vi "LR5_code.vi"(7 "data in":string, 8 "error in (no error)":errorcluster, 9 "Image Dst":T1) -> (0 "error out":errorcluster, 2 "data out":string)   [LabVIEW 2019]
uses:
  <vilib>/vision/Image Controls.llb/IMAQ Image.ctl
  Stage_var.vi
  Init_var.vi
  Color_num_var.vi
  Timer.vi
  Global_count_var.vi
  Camera_angle.vi
  Arm_stage_var.vi
  Mashina_podyehala.vi
  Ball_num_var.vi
  Completed_var.vi
  Sequence_var.vi
  Scanned.vi
  <vilib>/vision/NI_Vision_Development_Module.lvlib
  Simulated Robot/Simulation SubVIs/Simulation SubVIs.lvlib
panel:
  out "Left":dbl(slide)
  out "Right":dbl(slide) scale=0.0..1.0
  out "ForwR":dbl(slide) scale=0.0..1.0
  out "ForwL":dbl(slide) scale=0.0..1.0
  out "ForwardRight Distance (m)":dbl
  out "ForwardLeft Distance (m)":dbl
  out "Right Distance (m)":dbl
  out "Left Distance (m)":dbl
  in  "Start":bool
  out "Stage":u32
  out "Ball num":dbl
  out "Color now":dbl
  out "Arm stage":dbl
  out "Image":T1(plugin-control)
  out "Sequence":dbl[](array[numeric])
  out "Scanned":bool
  out "Completed":bool
  out "Performing...":u8(slide) scale=4.0..107.0
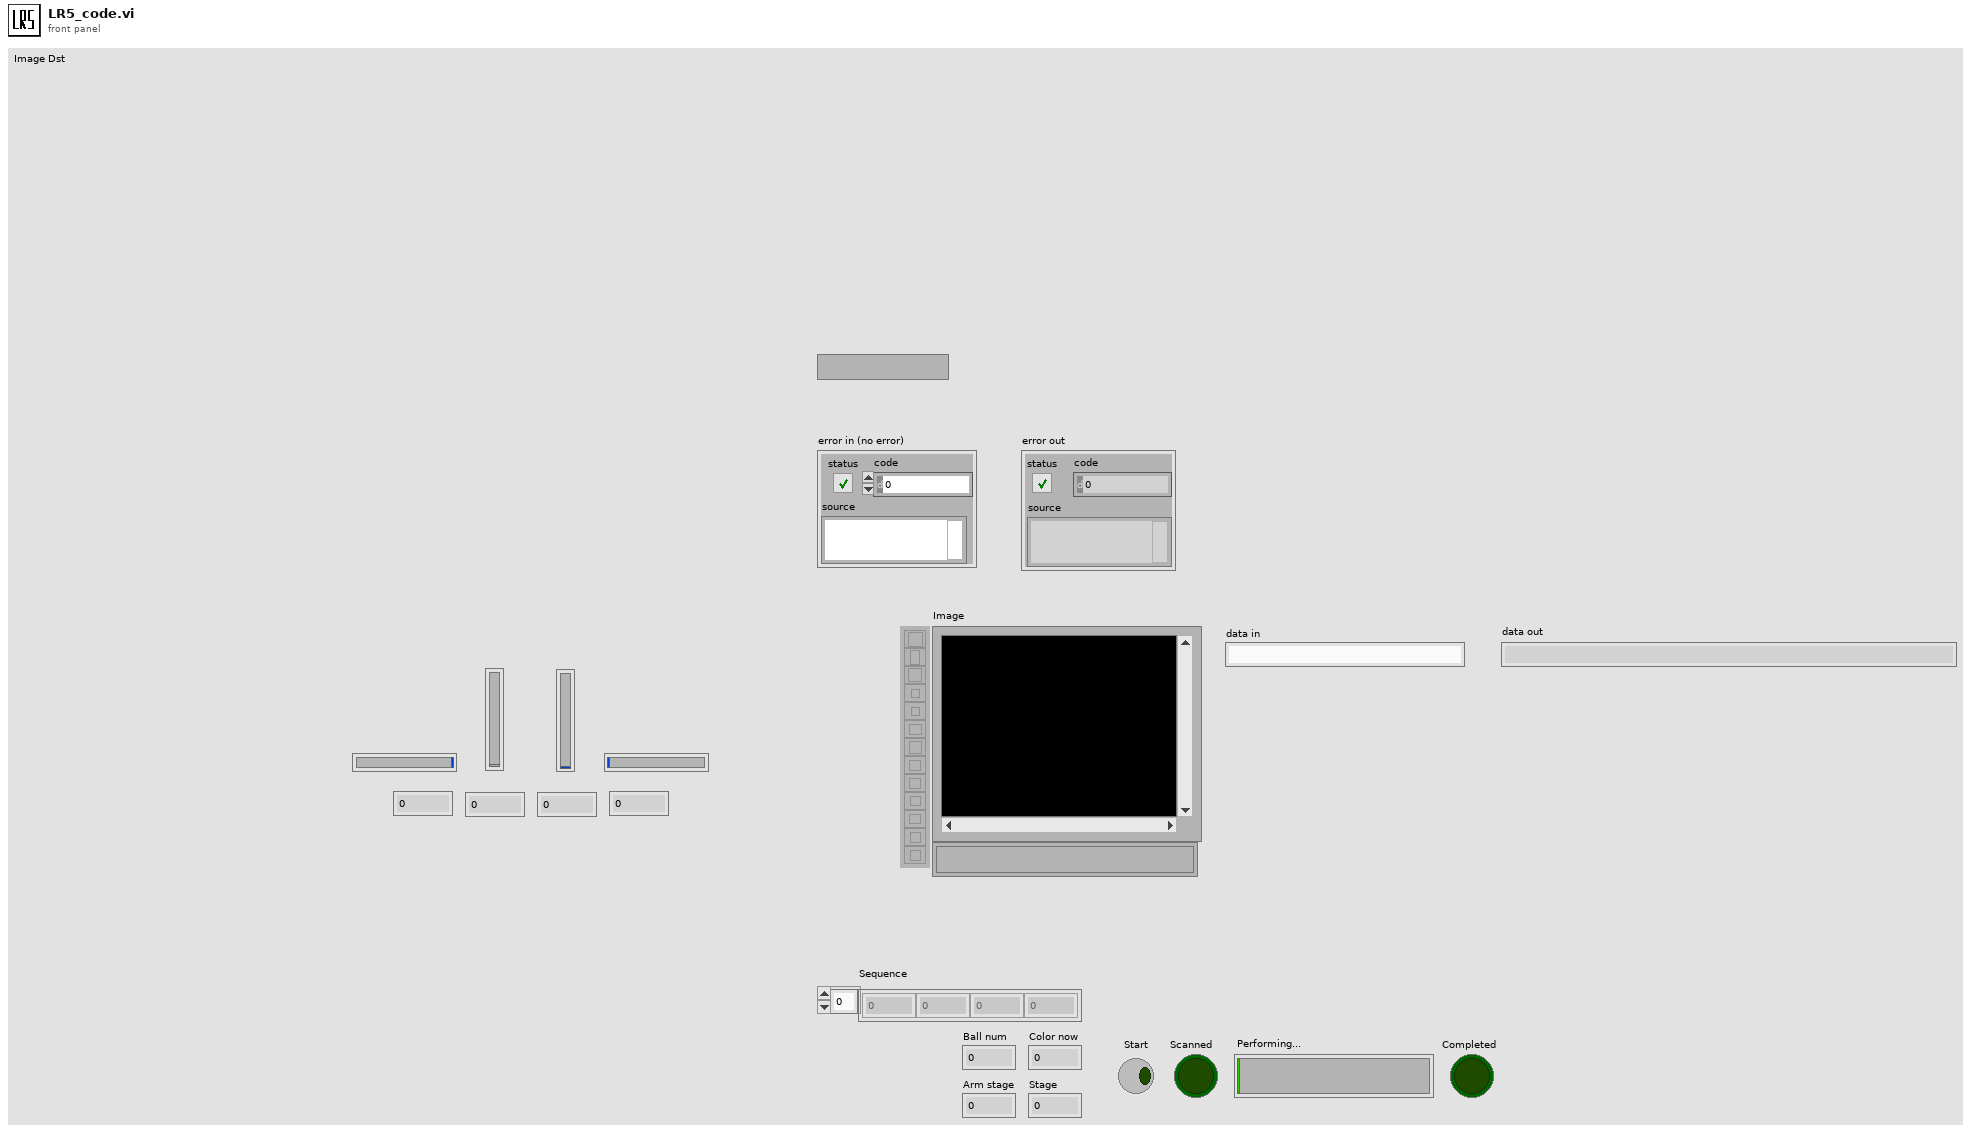
[diagram p1: front panel]
types:
  T1 = typedef "IMAQ Image.ctl" = refnum<image>
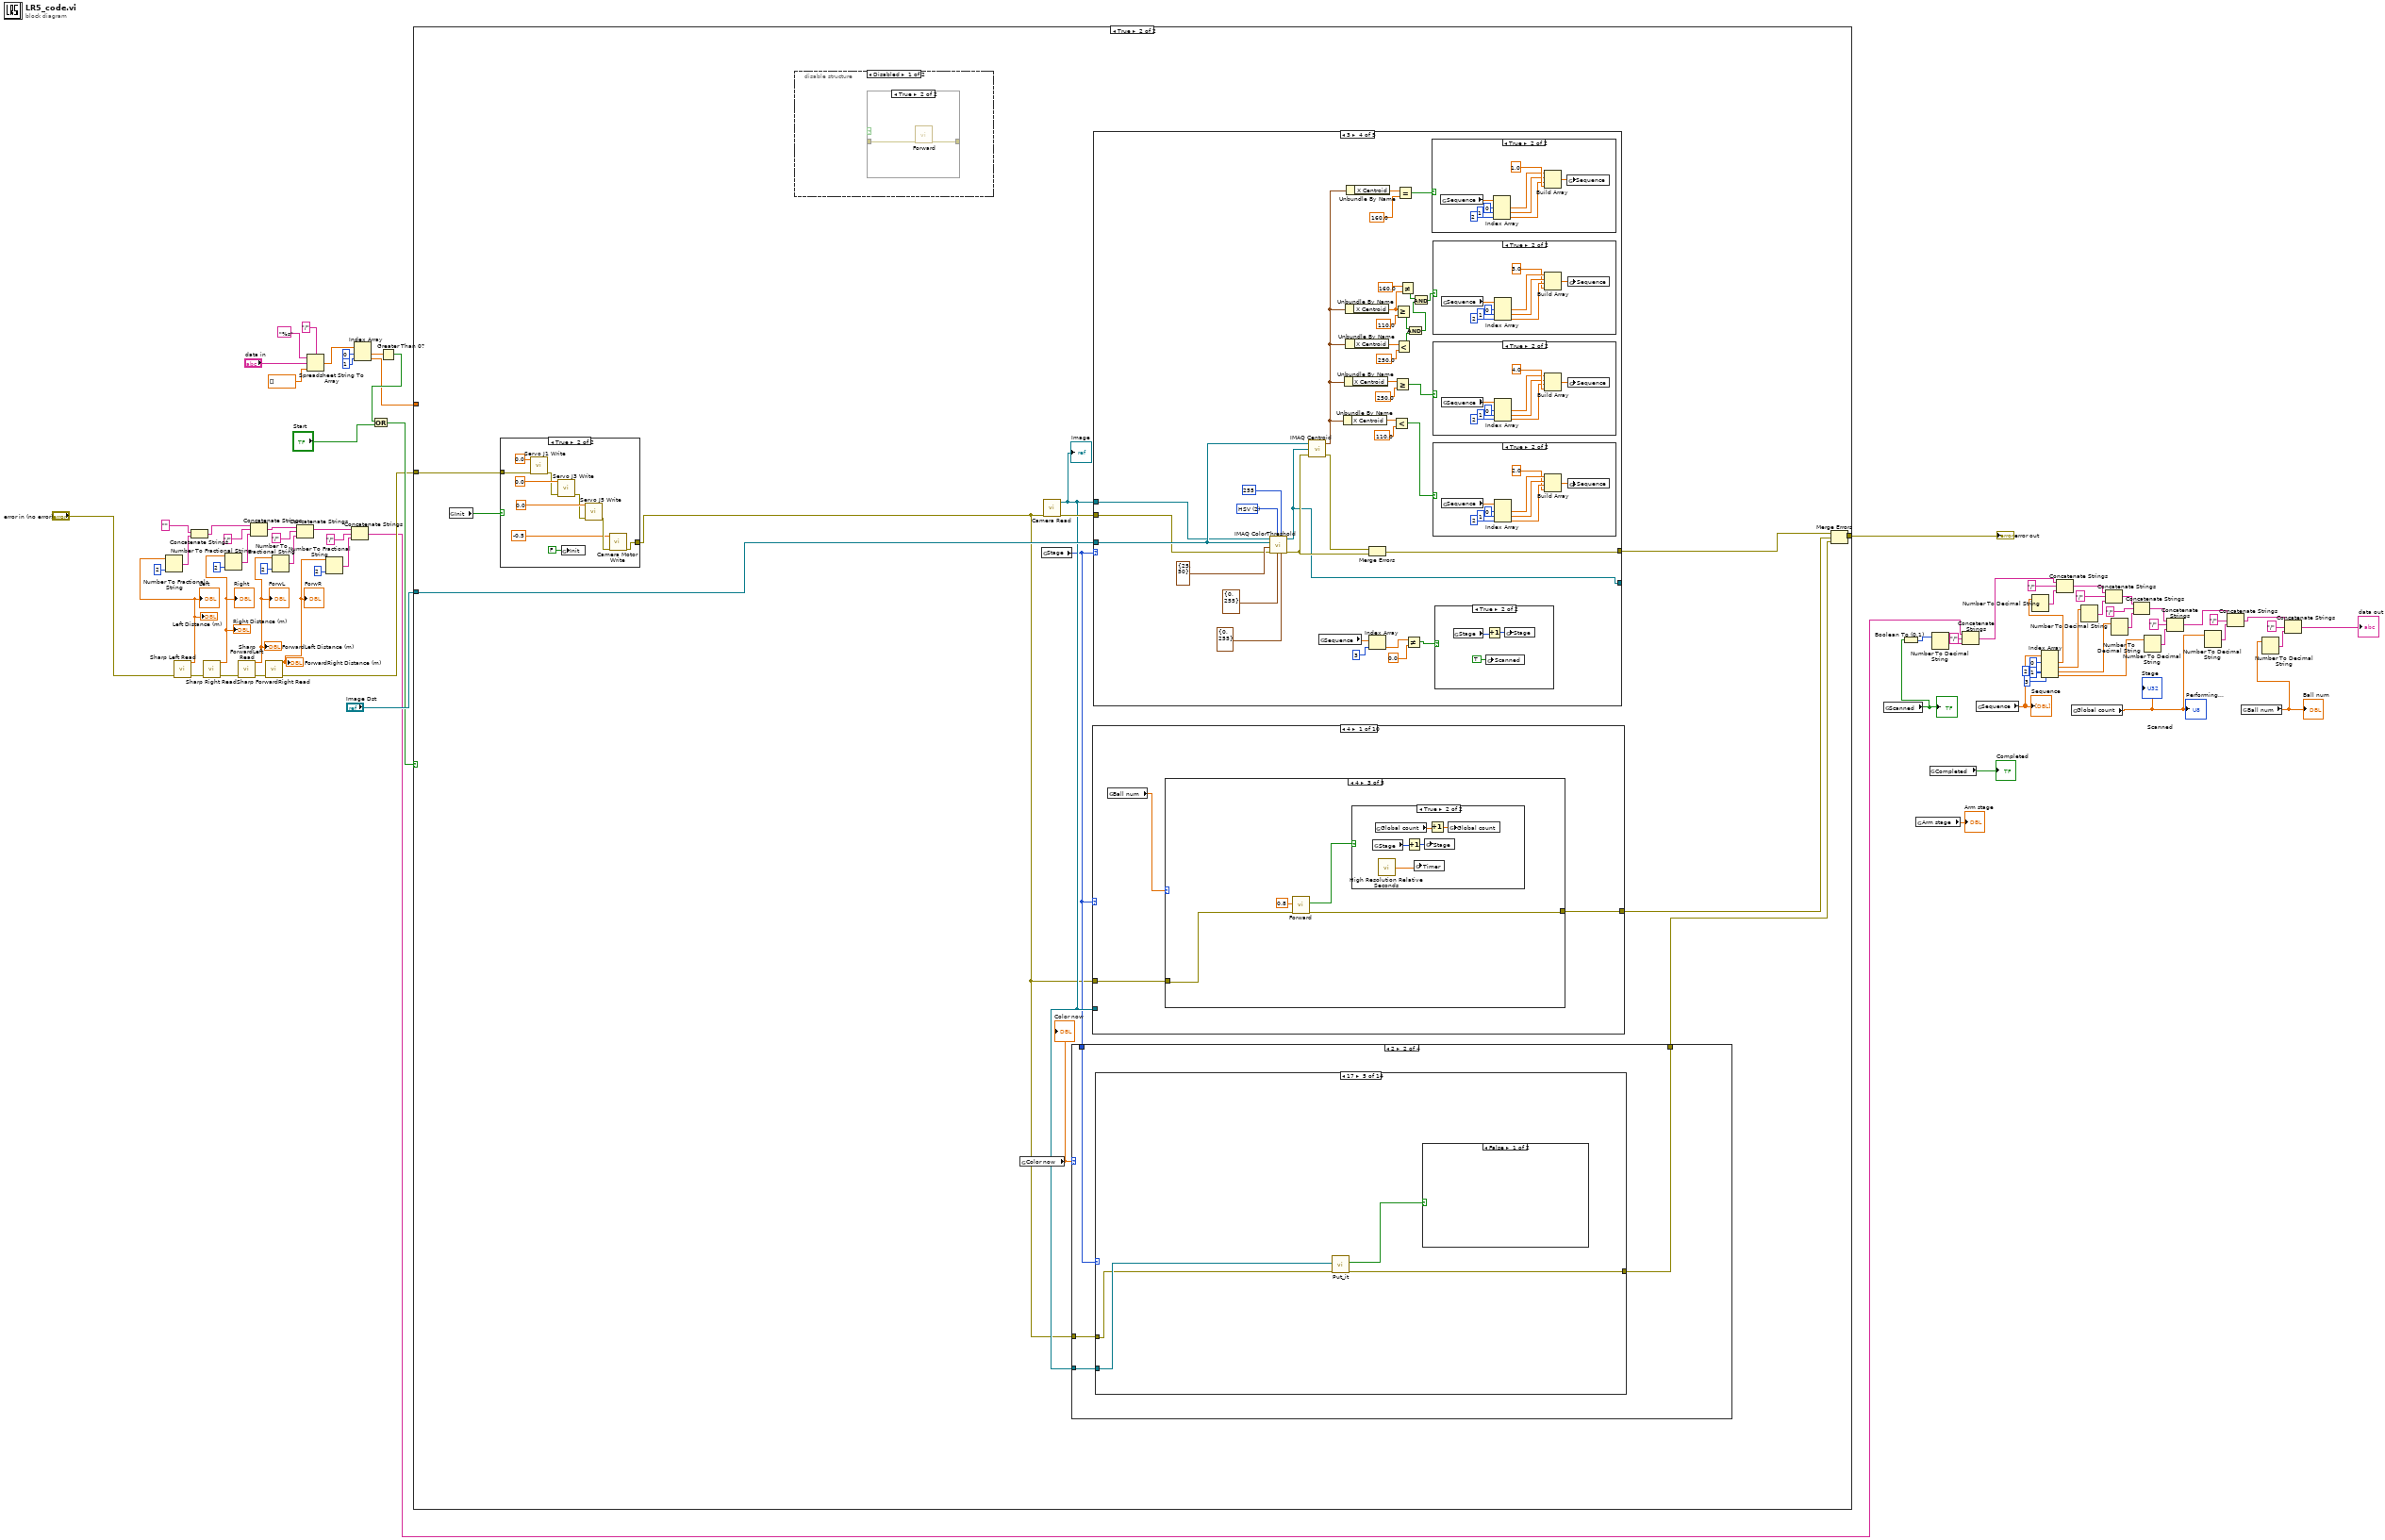
[diagram p0: block diagram]
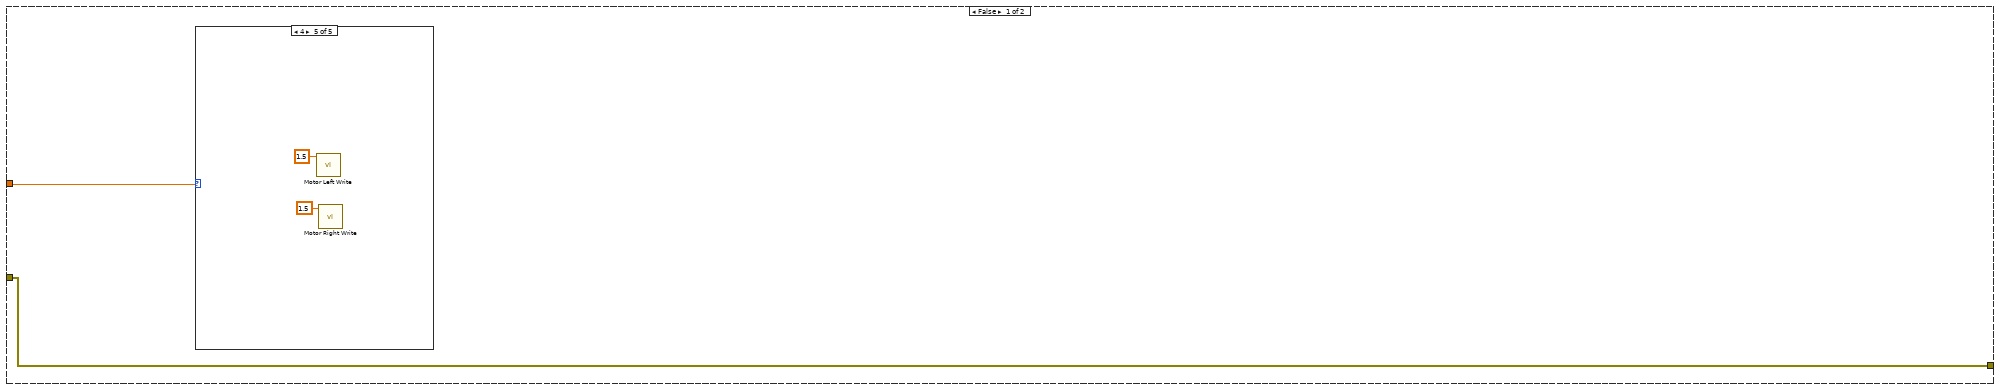
[diagram p2: hidden frame]
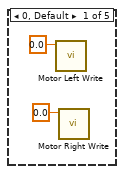
[diagram p3: hidden frame]
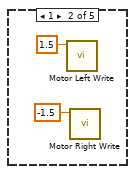
[diagram p4: hidden frame]
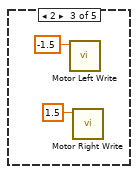
[diagram p5: hidden frame]
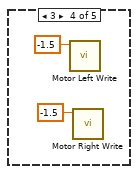
[diagram p6: hidden frame]
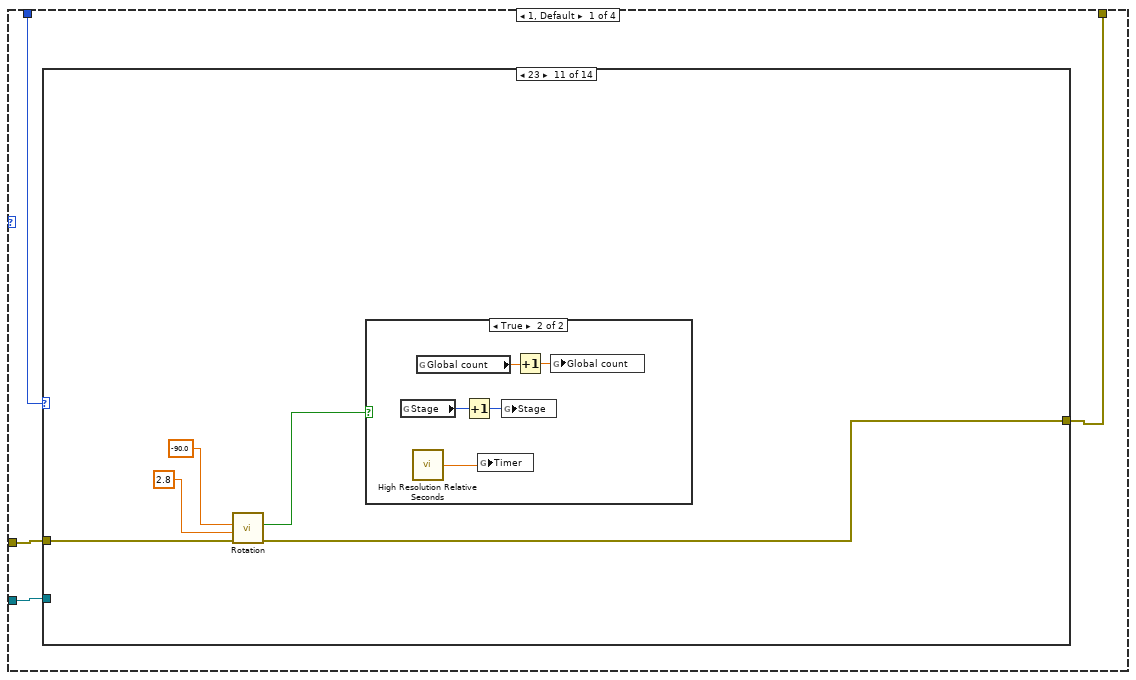
[diagram p7: hidden frame]
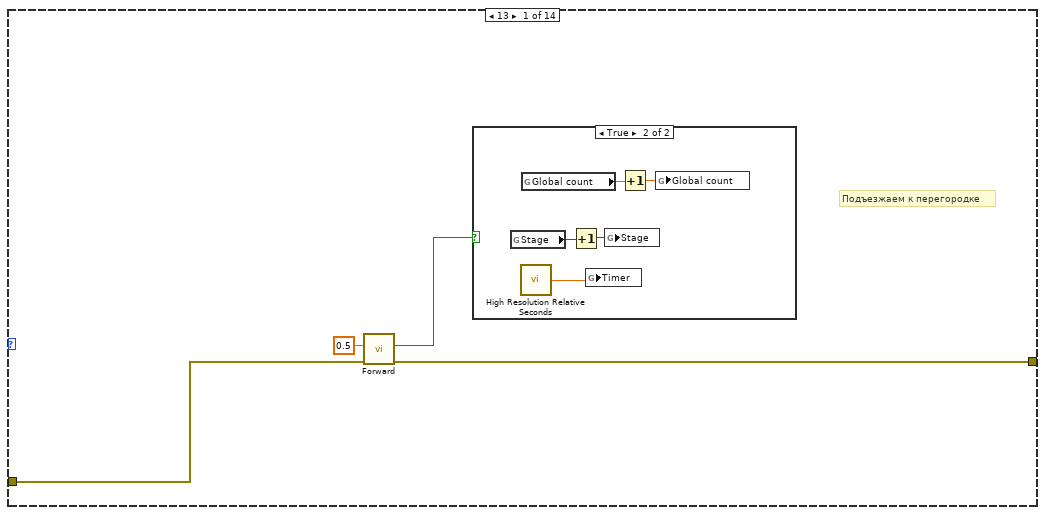
[diagram p8: hidden frame]
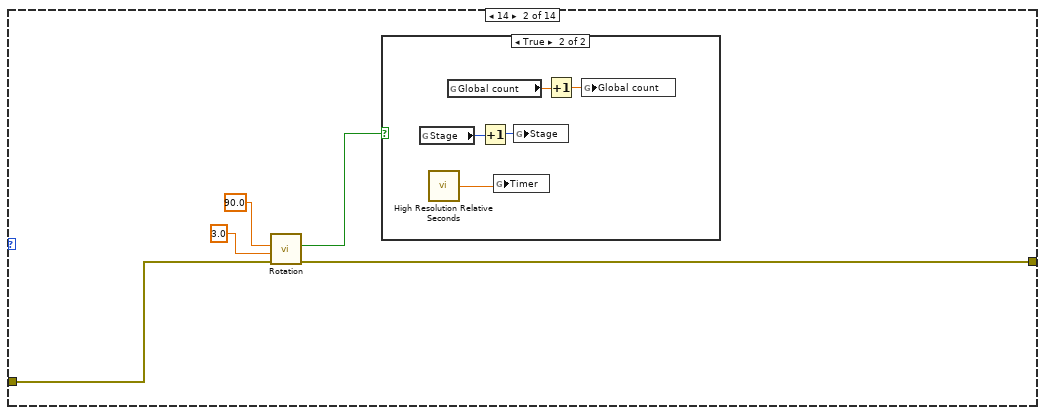
[diagram p10: hidden frame]
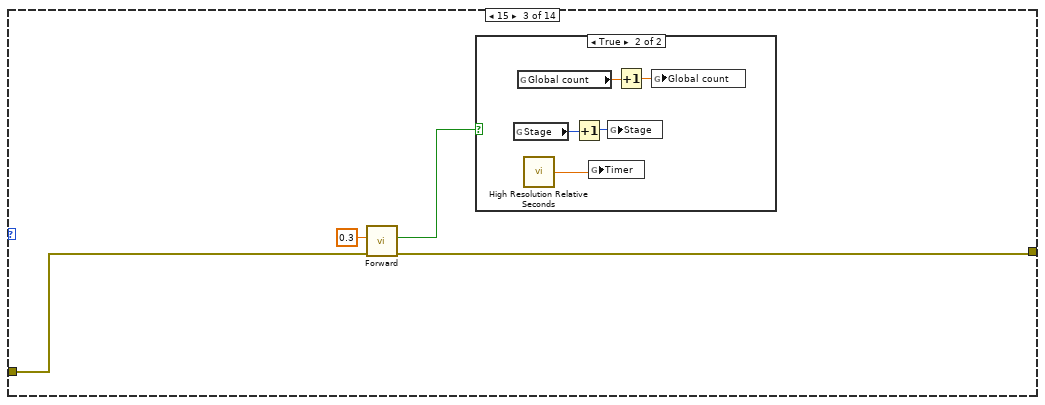
[diagram p12: hidden frame]
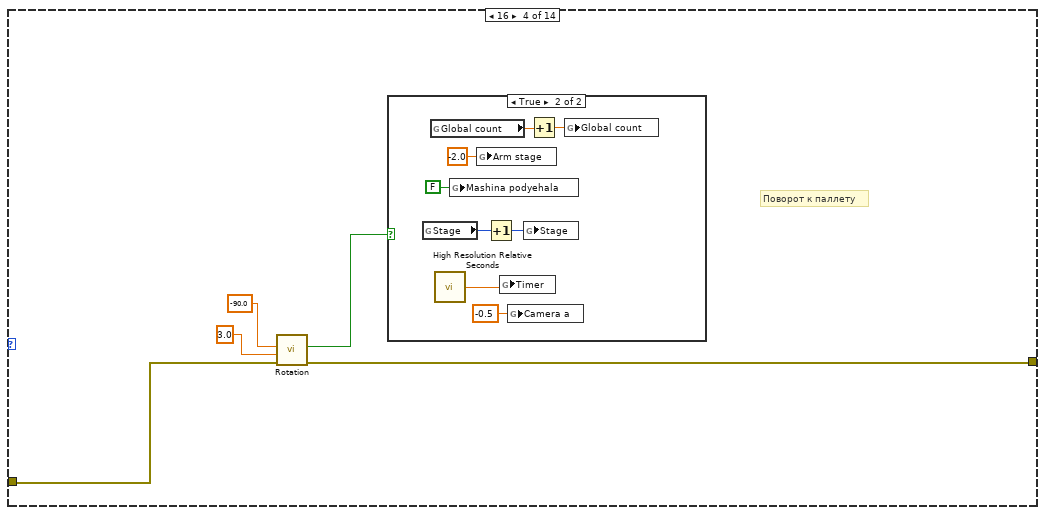
[diagram p14: hidden frame]
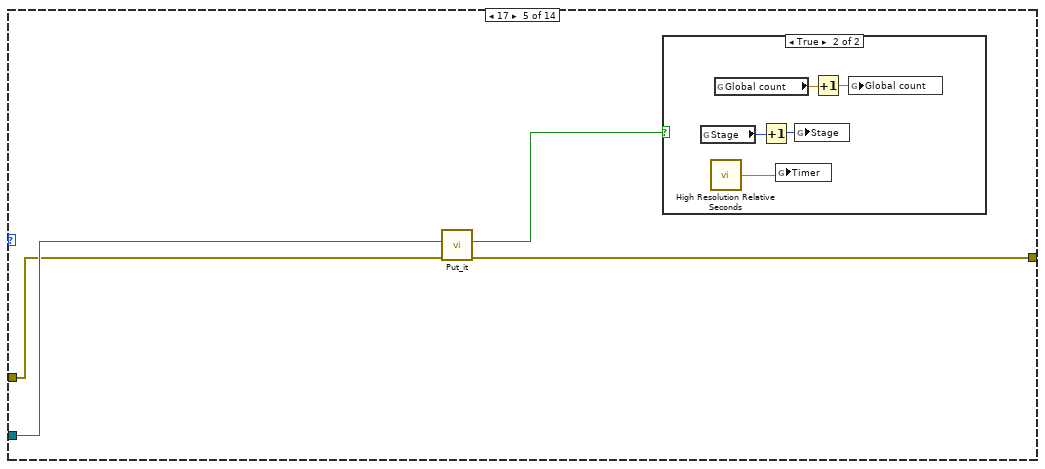
[diagram p16: hidden frame]
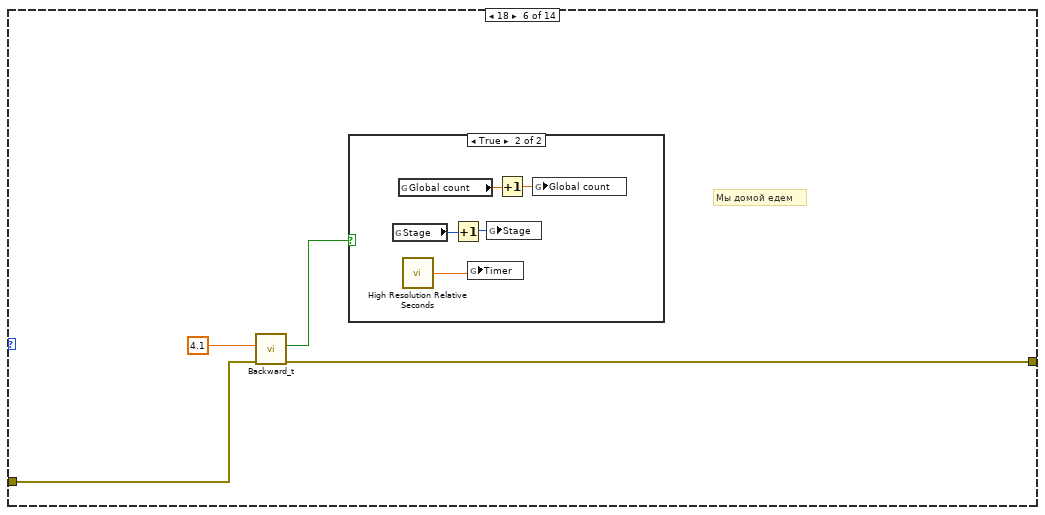
[diagram p18: hidden frame]
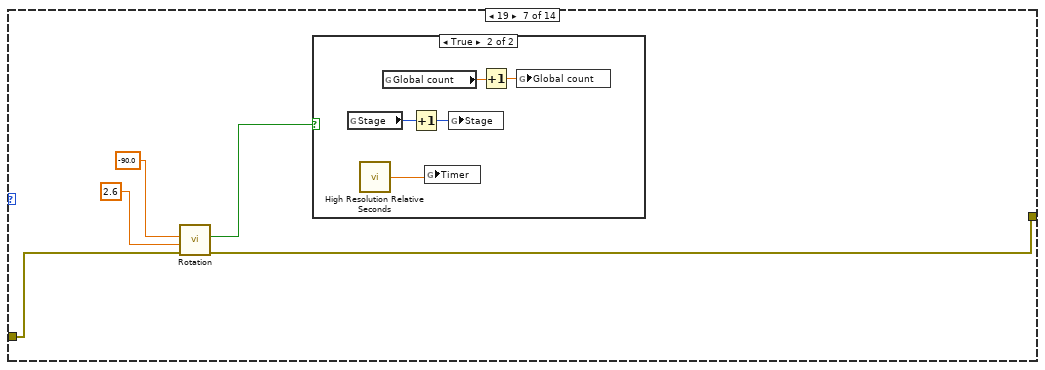
[diagram p20: hidden frame]
diagram:
  n1 = call "Sharp Left Read.vi"("error in (no error)"="error in (no error)") -> ("error out"=w59:errorcluster, "Left Distance (m)"=w52:dbl)  [unwired: 9 in]
  "Left Distance (m)" <- w52
  "Left" <- w52
  n2 = Number To Fractional String(number=w52, precision (6)=i16 2) -> (F-format string=w51:string)  [unwired: 2 in]
  n3 = Concatenate Strings("" ("string"), w51) -> (w41:string)
  n4 = call "Sharp Right Read.vi"("error in (no error)"=w59) -> ("error out"=w58:errorcluster, "Right Distance (m)"=w48:dbl)  [unwired: 9 in]
  "Right Distance (m)" <- w48
  "Right" <- w48
  n5 = Number To Fractional String(number=w48, precision (6)=i16 2) -> (F-format string=w50:string)  [unwired: 2 in]
  n6 = call "Sharp ForwardLeft Read.vi"("error in (no error)"=w58) -> ("error out"=w57:errorcluster, "ForwardLeft Distance (m)"=w45:dbl)  [unwired: 9 in]
  "ForwardLeft Distance (m)" <- w45
  "ForwL" <- w45
  n7 = Concatenate Strings(w41, "/" ("string"), w50) -> (w39:string)
  n8 = call "Sharp ForwardRight Read.vi"("error in (no error)"=w57) -> ("error out"=w55:errorcluster, "ForwardRight Distance (m)"=w42:dbl)  [unwired: 9 in]
  "ForwardRight Distance (m)" <- w42
  "ForwR" <- w42
  n9 = Number To Fractional String(number=w45, precision (6)=i16 2) -> (F-format string=w46:string)  [unwired: 2 in]
  n10 = Concatenate Strings(w39, "/" ("string"), w46) -> (w37:string)
  n11 = Spreadsheet String To Array(delimiter (Tab)="/", format string="%s", spreadsheet string="data in", array type (2D Dbl)=dbl[] []) -> (array=w71:dbl[])
  n12 = Number To Fractional String(number=w42, precision (6)=i16 2) -> (F-format string=w43:string)  [unwired: 2 in]
  n13 = Concatenate Strings(w37, "/" ("string"), w43) -> (w10:string)
  n14 = Index Array(array=w71, index #1=0 ("index"), index #2=1 ("index")) -> (element #1=w64:dbl, element #2=w62:dbl)
  n15 = Greater Than 0?(x=w64) -> (x > 0?=w63:bool)
  n16 = Or(x=w63, y="Start") -> (x .or. y?=w70:bool)
  n17 = case shown="True" w70 {
    tunnel: w55 -> [w77 w99]
    tunnel: [w77 w95] -> w75
    tunnel: "Image Dst" -> [_ w93]
    tunnel: w62 -> [w76 _]
    frame False {
      n18 = case shown="4" w76 {
        frame 0, Default {
          n19 = call "Motor Left Write.vi"("left motor ccw velocity (rad/s)"=0.0) -> ()  [unwired: 10 in, 1 out]
          n20 = call "Motor Right Write.vi"("right motor ccw velocity (rad/s)"=0.0) -> ()  [unwired: 10 in, 1 out]
        }
        frame 1 {
          n21 = call "Motor Left Write.vi"("left motor ccw velocity (rad/s)"=1.5) -> ()  [unwired: 10 in, 1 out]
          n22 = call "Motor Right Write.vi"("right motor ccw velocity (rad/s)"=-1.5) -> ()  [unwired: 10 in, 1 out]
        }
        frame 2 {
          n23 = call "Motor Left Write.vi"("left motor ccw velocity (rad/s)"=-1.5) -> ()  [unwired: 10 in, 1 out]
          n24 = call "Motor Right Write.vi"("right motor ccw velocity (rad/s)"=1.5) -> ()  [unwired: 10 in, 1 out]
        }
        frame 3 {
          n25 = call "Motor Left Write.vi"("left motor ccw velocity (rad/s)"=-1.5) -> ()  [unwired: 10 in, 1 out]
          n26 = call "Motor Right Write.vi"("right motor ccw velocity (rad/s)"=-1.5) -> ()  [unwired: 10 in, 1 out]
        }
        frame 4 {
          n27 = call "Motor Left Write.vi"("left motor ccw velocity (rad/s)"=1.5) -> ()  [unwired: 10 in, 1 out]
          n28 = call "Motor Right Write.vi"("right motor ccw velocity (rad/s)"=1.5) -> ()  [unwired: 10 in, 1 out]
        }
      }
    }
    frame True {
      n29 = global read "Init_var.vi" "Init"() -> (w98:bool)
      n30 = case shown="True" w98 {
        tunnel: w99 -> [w1006 w1009]
        tunnel: [w1006 w1007] -> w88
        frame False {
        }
        frame True {
          n31 = call "Servo J1 Write.vi"("error in (no error)"=w1009, "J1 Position (m)"=0.0) -> ("error out"=w1014:errorcluster)  [unwired: 9 in]
          n32 = call "Servo J3 Write.vi"("error in (no error)"=w1014, "J3 Position (m)"=0.0) -> ("error out"=w1013:errorcluster)  [unwired: 9 in]
          n33 = global write "Init_var.vi" "Init"(FALSE ("Init")) -> ()
          n34 = call "Servo J5 Write.vi"("error in (no error)"=w1013, "J5 Position (m)"=0.0) -> ("error out"=w1012:errorcluster)  [unwired: 9 in]
          n35 = call "Camera Motor Write.vi"("error in (no error)"=w1012, "Camera Position (rad)"=-0.5) -> ("error out"=w1007:errorcluster)  [unwired: 9 in]
        }
      }
      n36 = disable-structure shown="Disabled" {
        frame Disabled {
          n37 = case shown="True" w1321 {
            tunnel: [w1322 w1324] -> w1320
            tunnel: [w1322 w1323] -> _
            frame False {
            }
            frame True {
              n38 = call "Forward.vi"("error in (no error)"=w1324) -> ("error out"=w1323:errorcluster)  [unwired: 9 in, 1 out]
            }
          }
        }
        frame Enabled {
        }
      }
      n39 = global read "Color_num_var.vi" "Color now"() -> (w92:dbl)
      "Color now" <- w92
      n40 = global read "Stage_var.vi" "Stage"() -> (w90:u32)
      n41 = call "Camera Read.vi"("error in (no error)"=w88) -> ("error out"=w94:errorcluster, "Camera Image"=w91:T1)  [unwired: 9 in]
      "Image" <- w91
      n42 = case shown="2" w92 {
        tunnel: w88 -> [w102 w238 w373 w598]
        tunnel: w91 -> [w101 w237 w372 w597]
        tunnel: w90 -> [w100 w236 w371 w599]
        tunnel: [w103 w235 w370 w596] -> w89
        frame 1, Default {
          n43 = case shown="23" w100 {
            tunnel: w102 -> [w107 w117 w123 w133 w146 w157 w163 w176 w182 w192 w202 w212 w220 w234]
            tunnel: w101 -> [_ _ _ _ w148 _ _ _ _ _ _ _ _ _]
            tunnel: [w106 w116 w124 w132 w147 w156 w164 w175 w183 w193 w201 w211 w221 w234] -> w103
            frame 13 {
              # "Подъезжаем к перегородке"
              n44 = call "Forward.vi"("error in (no error)"=w107, "how close"=0.5) -> ("error out"=w106:errorcluster, "Done"=w104:bool)  [unwired: 8 in]
              n45 = case shown="True" w104 {
                frame False {
                }
                frame True {
                  n46 = global read "Stage_var.vi" "Stage"() -> (w112:u32)
                  n47 = call <vilib>:"High Resolution Relative Seconds.vi"() -> ("relative seconds"=w110:dbl)
                  n48 = global read "Global_count_var.vi" "Global count"() -> (w108:dbl)
                  n49 = Increment(x=w112) -> (x+1=w111:u32)
                  n50 = global write "Timer.vi" "Timer"(w110) -> ()
                  n51 = global write "Stage_var.vi" "Stage"(w111) -> ()
                  n52 = Increment(x=w108) -> (x+1=w109:dbl)
                  n53 = global write "Global_count_var.vi" "Global count"(w109) -> ()
                }
              }
            }
            frame 14 {
              n54 = call "Rotation.vi"("error in (no error)"=w117, "Time"=3.0, "Direction"=90.0 ("how close")) -> ("error out"=w116:errorcluster, "Done"=w115:bool)  [unwired: 7 in]
              n55 = case shown="True" w115 {
                frame False {
                }
                frame True {
                  n56 = global read "Stage_var.vi" "Stage"() -> (w122:u32)
                  n57 = call <vilib>:"High Resolution Relative Seconds.vi"() -> ("relative seconds"=w120:dbl)
                  n58 = global read "Global_count_var.vi" "Global count"() -> (w118:dbl)
                  n59 = Increment(x=w122) -> (x+1=w121:u32)
                  n60 = global write "Timer.vi" "Timer"(w120) -> ()
                  n61 = global write "Stage_var.vi" "Stage"(w121) -> ()
                  n62 = Increment(x=w118) -> (x+1=w119:dbl)
                  n63 = global write "Global_count_var.vi" "Global count"(w119) -> ()
                }
              }
            }
            frame 15 {
              n64 = call "Forward.vi"("error in (no error)"=w123, "how close"=0.3) -> ("error out"=w124:errorcluster, "Done"=w125:bool)  [unwired: 8 in]
              n65 = case shown="True" w125 {
                frame False {
                }
                frame True {
                  n66 = global read "Stage_var.vi" "Stage"() -> (w131:u32)
                  n67 = global read "Global_count_var.vi" "Global count"() -> (w127:dbl)
                  n68 = call <vilib>:"High Resolution Relative Seconds.vi"() -> ("relative seconds"=w129:dbl)
                  n69 = Increment(x=w131) -> (x+1=w130:u32)
                  n70 = global write "Timer.vi" "Timer"(w129) -> ()
                  n71 = global write "Stage_var.vi" "Stage"(w130) -> ()
                  n72 = Increment(x=w127) -> (x+1=w128:dbl)
                  n73 = global write "Global_count_var.vi" "Global count"(w128) -> ()
                }
              }
            }
            frame 16 {
              # "Поворот к паллету"
              n74 = call "Rotation.vi"("error in (no error)"=w133, "Time"=3.0, "Direction"=-90.0 ("how close")) -> ("error out"=w132:errorcluster, "Done"=w136:bool)  [unwired: 7 in]
              n75 = case shown="True" w136 {
                frame False {
                }
                frame True {
                  n76 = global read "Stage_var.vi" "Stage"() -> (w144:u32)
                  n77 = global read "Global_count_var.vi" "Global count"() -> (w137:dbl)
                  n78 = call <vilib>:"High Resolution Relative Seconds.vi"() -> ("relative seconds"=w142:dbl)
                  n79 = global write "Mashina_podyehala.vi" "Mashina podyehala"(FALSE ("Mashina podyehala")) -> ()
                  n80 = global write "Arm_stage_var.vi" "Arm stage"(-2.0 ("Arm stage")) -> ()
                  n81 = Increment(x=w144) -> (x+1=w143:u32)
                  n82 = global write "Timer.vi" "Timer"(w142) -> ()
                  n83 = global write "Camera_angle.vi" "Camera a"(-0.5 ("Camera a")) -> ()
                  n84 = global write "Stage_var.vi" "Stage"(w143) -> ()
                  n85 = Increment(x=w137) -> (x+1=w138:dbl)
                  n86 = global write "Global_count_var.vi" "Global count"(w138) -> ()
                }
              }
            }
            frame 17 {
              n87 = call "Put_it.vi"("error in (no error) 2"=w146, "Camera Image"=w148) -> ("error out"=w147:errorcluster, "Done"=w145:bool)  [unwired: 8 in]
              n88 = case shown="True" w145 {
                frame False {
                }
                frame True {
                  n89 = global read "Stage_var.vi" "Stage"() -> (w153:u32)
                  n90 = call <vilib>:"High Resolution Relative Seconds.vi"() -> ("relative seconds"=w151:dbl)
                  n91 = global read "Global_count_var.vi" "Global count"() -> (w149:dbl)
                  n92 = Increment(x=w153) -> (x+1=w152:u32)
                  n93 = global write "Timer.vi" "Timer"(w151) -> ()
                  n94 = global write "Stage_var.vi" "Stage"(w152) -> ()
                  n95 = Increment(x=w149) -> (x+1=w150:dbl)
                  n96 = global write "Global_count_var.vi" "Global count"(w150) -> ()
                }
              }
            }
            frame 18 {
              # "Мы домой едем"
              n97 = call "Backward_t.vi"("error in (no error)"=w157, "Time"=4.1 ("how close")) -> ("error out"=w156:errorcluster, "Done"=w155:bool)  [unwired: 8 in]
              n98 = case shown="True" w155 {
                frame False {
                }
                frame True {
                  n99 = global read "Stage_var.vi" "Stage"() -> (w162:u32)
                  n100 = global read "Global_count_var.vi" "Global count"() -> (w158:dbl)
                  n101 = call <vilib>:"High Resolution Relative Seconds.vi"() -> ("relative seconds"=w160:dbl)
                  n102 = Increment(x=w162) -> (x+1=w161:u32)
                  n103 = global write "Timer.vi" "Timer"(w160) -> ()
                  n104 = global write "Stage_var.vi" "Stage"(w161) -> ()
                  n105 = Increment(x=w158) -> (x+1=w159:dbl)
                  n106 = global write "Global_count_var.vi" "Global count"(w159) -> ()
                }
              }
            }
            frame 19 {
              n107 = call "Rotation.vi"("error in (no error)"=w163, "Time"=2.6, "Direction"=-90.0 ("how close")) -> ("error out"=w164:errorcluster, "Done"=w167:bool)  [unwired: 7 in]
              n108 = case shown="True" w167 {
                frame False {
                }
                frame True {
                  n109 = global read "Stage_var.vi" "Stage"() -> (w172:u32)
                  n110 = call <vilib>:"High Resolution Relative Seconds.vi"() -> ("relative seconds"=w170:dbl)
                  n111 = global read "Global_count_var.vi" "Global count"() -> (w168:dbl)
                  n112 = Increment(x=w172) -> (x+1=w171:u32)
                  n113 = global write "Timer.vi" "Timer"(w170) -> ()
                  n114 = global write "Stage_var.vi" "Stage"(w171) -> ()
                  n115 = Increment(x=w168) -> (x+1=w169:dbl)
                  n116 = global write "Global_count_var.vi" "Global count"(w169) -> ()
                }
              }
            }
            frame 20 {
              n117 = call "Forward_t.vi"("error in (no error)"=w176, "Time"=5.0 ("how close")) -> ("error out"=w175:errorcluster, "Done"=w173:bool)  [unwired: 8 in]
              n118 = case shown="True" w173 {
                frame False {
                }
                frame True {
                  n119 = global read "Stage_var.vi" "Stage"() -> (w181:u32)
                  n120 = call <vilib>:"High Resolution Relative Seconds.vi"() -> ("relative seconds"=w179:dbl)
                  n121 = global read "Global_count_var.vi" "Global count"() -> (w177:dbl)
                  n122 = Increment(x=w181) -> (x+1=w180:u32)
                  n123 = global write "Timer.vi" "Timer"(w179) -> ()
                  n124 = global write "Stage_var.vi" "Stage"(w180) -> ()
                  n125 = Increment(x=w177) -> (x+1=w178:dbl)
                  n126 = global write "Global_count_var.vi" "Global count"(w178) -> ()
                }
              }
            }
            frame 21 {
              n127 = call "Rotation.vi"("error in (no error)"=w182, "Time"=2.7, "Direction"=-90.0 ("how close")) -> ("error out"=w183:errorcluster, "Done"=w186:bool)  [unwired: 7 in]
              n128 = case shown="True" w186 {
                frame False {
                }
                frame True {
                  n129 = global read "Stage_var.vi" "Stage"() -> (w191:u32)
                  n130 = call <vilib>:"High Resolution Relative Seconds.vi"() -> ("relative seconds"=w189:dbl)
                  n131 = global read "Global_count_var.vi" "Global count"() -> (w187:dbl)
                  n132 = Increment(x=w191) -> (x+1=w190:u32)
                  n133 = global write "Timer.vi" "Timer"(w189) -> ()
                  n134 = global write "Stage_var.vi" "Stage"(w190) -> ()
                  n135 = Increment(x=w187) -> (x+1=w188:dbl)
                  n136 = global write "Global_count_var.vi" "Global count"(w188) -> ()
                }
              }
            }
            frame 22 {
              n137 = call "Forward.vi"("error in (no error)"=w192, "how close"=0.18) -> ("error out"=w193:errorcluster, "Done"=w194:bool)  [unwired: 8 in]
              n138 = case shown="True" w194 {
                frame False {
                }
                frame True {
                  n139 = global read "Stage_var.vi" "Stage"() -> (w200:u32)
                  n140 = global read "Global_count_var.vi" "Global count"() -> (w196:dbl)
                  n141 = call <vilib>:"High Resolution Relative Seconds.vi"() -> ("relative seconds"=w198:dbl)
                  n142 = Increment(x=w200) -> (x+1=w199:u32)
                  n143 = global write "Timer.vi" "Timer"(w198) -> ()
                  n144 = global write "Stage_var.vi" "Stage"(w199) -> ()
                  n145 = Increment(x=w196) -> (x+1=w197:dbl)
                  n146 = global write "Global_count_var.vi" "Global count"(w197) -> ()
                }
              }
            }
            frame 23 {
              n147 = call "Rotation.vi"("error in (no error)"=w202, "Time"=2.8, "Direction"=-90.0 ("how close")) -> ("error out"=w201:errorcluster, "Done"=w205:bool)  [unwired: 7 in]
              n148 = case shown="True" w205 {
                frame False {
                }
                frame True {
                  n149 = global read "Stage_var.vi" "Stage"() -> (w210:u32)
                  n150 = call <vilib>:"High Resolution Relative Seconds.vi"() -> ("relative seconds"=w208:dbl)
                  n151 = global read "Global_count_var.vi" "Global count"() -> (w206:dbl)
                  n152 = Increment(x=w210) -> (x+1=w209:u32)
                  n153 = global write "Timer.vi" "Timer"(w208) -> ()
                  n154 = global write "Stage_var.vi" "Stage"(w209) -> ()
                  n155 = Increment(x=w206) -> (x+1=w207:dbl)
                  n156 = global write "Global_count_var.vi" "Global count"(w207) -> ()
                }
              }
            }
            frame 24 {
              # "Финишная"
              n157 = call "Forward.vi"("error in (no error)"=w212, "how close"=0.47) -> ("error out"=w211:errorcluster, "Done"=w213:bool)  [unwired: 8 in]
              n158 = case shown="True" w213 {
                frame False {
                }
                frame True {
                  n159 = global read "Stage_var.vi" "Stage"() -> (w219:u32)
                  n160 = global read "Global_count_var.vi" "Global count"() -> (w215:dbl)
                  n161 = call <vilib>:"High Resolution Relative Seconds.vi"() -> ("relative seconds"=w217:dbl)
                  n162 = Increment(x=w219) -> (x+1=w218:u32)
                  n163 = global write "Timer.vi" "Timer"(w217) -> ()
                  n164 = global write "Stage_var.vi" "Stage"(w218) -> ()
                  n165 = Increment(x=w215) -> (x+1=w216:dbl)
                  n166 = global write "Global_count_var.vi" "Global count"(w216) -> ()
                }
              }
            }
            frame 25 {
              # "R"
              # "Поворот на лотки"
              n167 = call "Rotation.vi"("error in (no error)"=w220, "Time"=2.6, "Direction"=-90.0 ("how close")) -> ("error out"=w221:errorcluster, "Done"=w224:bool)  [unwired: 7 in]
              n168 = case shown="True" w224 {
                frame False {
                }
                frame True {
                  n169 = global read "Ball_num_var.vi" "Ball num"() -> (w232:dbl)
                  n170 = call <vilib>:"High Resolution Relative Seconds.vi"() -> ("relative seconds"=w233:dbl)
                  n171 = global read "Global_count_var.vi" "Global count"() -> (w225:dbl)
                  n172 = global write "Stage_var.vi" "Stage"(u32 4 ("Stage")) -> ()
                  n173 = Increment(x=w232) -> (x+1=w231:dbl)
                  n174 = global write "Timer.vi" "Timer"(w233) -> ()
                  n175 = global write "Ball_num_var.vi" "Ball num"(w231) -> ()
                  n176 = Increment(x=w225) -> (x+1=w226:dbl)
                  n177 = global write "Global_count_var.vi" "Global count"(w226) -> ()
                  n178 = global write "Mashina_podyehala.vi" "Mashina podyehala"(FALSE ("Mashina podyehala")) -> ()
                  n179 = global write "Camera_angle.vi" "Camera a"(-0.7 ("Camera a")) -> ()
                  n180 = global write "Arm_stage_var.vi" "Arm stage"(-2.0 ("Arm stage")) -> ()
                }
              }
            }
            frame Default {
            }
          }
        }
        frame 2 {
          n181 = case shown="17" w236 {
            tunnel: w238 -> [w242 w252 w261 w268 w281 w292 w298 w311 w317 w327 w337 w347 w357 w369]
            tunnel: w237 -> [_ _ _ _ w283 _ _ _ _ _ _ _ _ _]
            tunnel: [w241 w251 w260 w267 w282 w291 w299 w310 w318 w328 w336 w346 w356 w369] -> w235
            frame 13 {
              # "Подъезжаем к перегородке"
              n182 = call "Forward.vi"("error in (no error)"=w242, "how close"=0.5) -> ("error out"=w241:errorcluster, "Done"=w239:bool)  [unwired: 8 in]
              n183 = case shown="True" w239 {
                frame False {
                }
                frame True {
                  n184 = global read "Stage_var.vi" "Stage"() -> (w247:u32)
                  n185 = global read "Global_count_var.vi" "Global count"() -> (w243:dbl)
                  n186 = call <vilib>:"High Resolution Relative Seconds.vi"() -> ("relative seconds"=w245:dbl)
                  n187 = Increment(x=w247) -> (x+1=w246:u32)
                  n188 = global write "Timer.vi" "Timer"(w245) -> ()
                  n189 = global write "Stage_var.vi" "Stage"(w246) -> ()
                  n190 = Increment(x=w243) -> (x+1=w244:dbl)
                  n191 = global write "Global_count_var.vi" "Global count"(w244) -> ()
                }
              }
            }
            frame 14 {
              n192 = call "Rotation.vi"("error in (no error)"=w252, "Time"=3.0, "Direction"=-90.0 ("how close")) -> ("error out"=w251:errorcluster, "Done"=w250:bool)  [unwired: 7 in]
              n193 = case shown="True" w250 {
                frame False {
                }
                frame True {
                  n194 = global read "Stage_var.vi" "Stage"() -> (w257:u32)
                  n195 = call <vilib>:"High Resolution Relative Seconds.vi"() -> ("relative seconds"=w255:dbl)
                  n196 = global read "Global_count_var.vi" "Global count"() -> (w253:dbl)
                  n197 = Increment(x=w257) -> (x+1=w256:u32)
                  n198 = global write "Timer.vi" "Timer"(w255) -> ()
                  n199 = global write "Stage_var.vi" "Stage"(w256) -> ()
                  n200 = Increment(x=w253) -> (x+1=w254:dbl)
                  n201 = global write "Global_count_var.vi" "Global count"(w254) -> ()
                }
              }
            }
            frame 15 {
              # "G"
              n202 = call "Forward_t.vi"("error in (no error)"=w261, "Time"=4.5 ("how close")) -> ("error out"=w260:errorcluster, "Done"=w259:bool)  [unwired: 8 in]
              n203 = case shown="True" w259 {
                frame False {
                }
                frame True {
                  n204 = global read "Global_count_var.vi" "Global count"() -> (w262:dbl)
                  n205 = global read "Stage_var.vi" "Stage"() -> (w266:u32)
                  n206 = call <vilib>:"High Resolution Relative Seconds.vi"() -> ("relative seconds"=w264:dbl)
                  n207 = Increment(x=w266) -> (x+1=w265:u32)
                  n208 = global write "Timer.vi" "Timer"(w264) -> ()
                  n209 = global write "Stage_var.vi" "Stage"(w265) -> ()
                  n210 = Increment(x=w262) -> (x+1=w263:dbl)
                  n211 = global write "Global_count_var.vi" "Global count"(w263) -> ()
                }
              }
            }
            frame 16 {
              # "Поворот к паллету"
              n212 = call "Rotation.vi"("error in (no error)"=w268, "Time"=3.0, "Direction"=90.0 ("how close")) -> ("error out"=w267:errorcluster, "Done"=w271:bool)  [unwired: 7 in]
              n213 = case shown="True" w271 {
                frame False {
                }
                frame True {
                  n214 = global read "Stage_var.vi" "Stage"() -> (w279:u32)
                  n215 = global read "Global_count_var.vi" "Global count"() -> (w272:dbl)
                  n216 = call <vilib>:"High Resolution Relative Seconds.vi"() -> ("relative seconds"=w277:dbl)
                  n217 = global write "Mashina_podyehala.vi" "Mashina podyehala"(FALSE ("Mashina podyehala")) -> ()
                  n218 = global write "Arm_stage_var.vi" "Arm stage"(-2.0 ("Arm stage")) -> ()
                  n219 = Increment(x=w279) -> (x+1=w278:u32)
                  n220 = global write "Timer.vi" "Timer"(w277) -> ()
                  n221 = global write "Camera_angle.vi" "Camera a"(-0.5 ("Camera a")) -> ()
                  n222 = global write "Stage_var.vi" "Stage"(w278) -> ()
                  n223 = Increment(x=w272) -> (x+1=w273:dbl)
                  n224 = global write "Global_count_var.vi" "Global count"(w273) -> ()
                }
              }
            }
            frame 17 {
              n225 = call "Put_it.vi"("error in (no error) 2"=w281, "Camera Image"=w283) -> ("error out"=w282:errorcluster, "Done"=w280:bool)  [unwired: 8 in]
              n226 = case shown="False" w280 {
                frame False {
                }
                frame True {
                  n227 = global read "Global_count_var.vi" "Global count"() -> (w284:dbl)
                  n228 = global read "Stage_var.vi" "Stage"() -> (w288:u32)
                  n229 = call <vilib>:"High Resolution Relative Seconds.vi"() -> ("relative seconds"=w286:dbl)
                  n230 = Increment(x=w288) -> (x+1=w287:u32)
                  n231 = global write "Timer.vi" "Timer"(w286) -> ()
                  n232 = global write "Stage_var.vi" "Stage"(w287) -> ()
                  n233 = Increment(x=w284) -> (x+1=w285:dbl)
                  n234 = global write "Global_count_var.vi" "Global count"(w285) -> ()
                }
              }
            }
            frame 18 {
              # "Мы домой едем"
              n235 = call "Backward_t.vi"("error in (no error)"=w292, "Time"=3.0 ("how close")) -> ("error out"=w291:errorcluster, "Done"=w290:bool)  [unwired: 8 in]
              n236 = case shown="True" w290 {
                frame False {
                }
                frame True {
                  n237 = global read "Stage_var.vi" "Stage"() -> (w297:u32)
                  n238 = global read "Global_count_var.vi" "Global count"() -> (w293:dbl)
                  n239 = call <vilib>:"High Resolution Relative Seconds.vi"() -> ("relative seconds"=w295:dbl)
                  n240 = Increment(x=w297) -> (x+1=w296:u32)
                  n241 = global write "Timer.vi" "Timer"(w295) -> ()
                  n242 = global write "Stage_var.vi" "Stage"(w296) -> ()
                  n243 = Increment(x=w293) -> (x+1=w294:dbl)
                  n244 = global write "Global_count_var.vi" "Global count"(w294) -> ()
                }
              }
            }
            frame 19 {
              n245 = call "Rotation.vi"("error in (no error)"=w298, "Time"=3.5, "Direction"=90.0 ("how close")) -> ("error out"=w299:errorcluster, "Done"=w302:bool)  [unwired: 7 in]
              n246 = case shown="True" w302 {
                frame False {
                }
                frame True {
                  n247 = global read "Stage_var.vi" "Stage"() -> (w307:u32)
                  n248 = call <vilib>:"High Resolution Relative Seconds.vi"() -> ("relative seconds"=w305:dbl)
                  n249 = global read "Global_count_var.vi" "Global count"() -> (w303:dbl)
                  n250 = Increment(x=w307) -> (x+1=w306:u32)
                  n251 = global write "Timer.vi" "Timer"(w305) -> ()
                  n252 = global write "Stage_var.vi" "Stage"(w306) -> ()
                  n253 = Increment(x=w303) -> (x+1=w304:dbl)
                  n254 = global write "Global_count_var.vi" "Global count"(w304) -> ()
                }
              }
            }
            frame 20 {
              n255 = call "Forward_t.vi"("error in (no error)"=w311, "Time"=5.0 ("how close")) -> ("error out"=w310:errorcluster, "Done"=w308:bool)  [unwired: 8 in]
              n256 = case shown="True" w308 {
                frame False {
                }
                frame True {
                  n257 = global read "Stage_var.vi" "Stage"() -> (w316:u32)
                  n258 = call <vilib>:"High Resolution Relative Seconds.vi"() -> ("relative seconds"=w314:dbl)
                  n259 = global read "Global_count_var.vi" "Global count"() -> (w312:dbl)
                  n260 = Increment(x=w316) -> (x+1=w315:u32)
                  n261 = global write "Timer.vi" "Timer"(w314) -> ()
                  n262 = global write "Stage_var.vi" "Stage"(w315) -> ()
                  n263 = Increment(x=w312) -> (x+1=w313:dbl)
                  n264 = global write "Global_count_var.vi" "Global count"(w313) -> ()
                }
              }
            }
            frame 21 {
              n265 = call "Rotation.vi"("error in (no error)"=w317, "Time"=2.3, "Direction"=90.0 ("how close")) -> ("error out"=w318:errorcluster, "Done"=w321:bool)  [unwired: 7 in]
              n266 = case shown="True" w321 {
                frame False {
                }
                frame True {
                  n267 = global read "Stage_var.vi" "Stage"() -> (w326:u32)
                  n268 = call <vilib>:"High Resolution Relative Seconds.vi"() -> ("relative seconds"=w324:dbl)
                  n269 = global read "Global_count_var.vi" "Global count"() -> (w322:dbl)
                  n270 = Increment(x=w326) -> (x+1=w325:u32)
                  n271 = global write "Timer.vi" "Timer"(w324) -> ()
                  n272 = global write "Stage_var.vi" "Stage"(w325) -> ()
                  n273 = Increment(x=w322) -> (x+1=w323:dbl)
                  n274 = global write "Global_count_var.vi" "Global count"(w323) -> ()
                }
              }
            }
            frame 22 {
              n275 = call "Forward.vi"("error in (no error)"=w327, "how close"=0.18) -> ("error out"=w328:errorcluster, "Done"=w329:bool)  [unwired: 8 in]
              n276 = case shown="True" w329 {
                frame False {
                }
                frame True {
                  n277 = global read "Stage_var.vi" "Stage"() -> (w335:u32)
                  n278 = call <vilib>:"High Resolution Relative Seconds.vi"() -> ("relative seconds"=w333:dbl)
                  n279 = global read "Global_count_var.vi" "Global count"() -> (w331:dbl)
                  n280 = Increment(x=w335) -> (x+1=w334:u32)
                  n281 = global write "Timer.vi" "Timer"(w333) -> ()
                  n282 = global write "Stage_var.vi" "Stage"(w334) -> ()
                  n283 = Increment(x=w331) -> (x+1=w332:dbl)
                  n284 = global write "Global_count_var.vi" "Global count"(w332) -> ()
                }
              }
            }
            frame 23 {
              n285 = call "Rotation.vi"("error in (no error)"=w337, "Time"=2.8, "Direction"=-90.0 ("how close")) -> ("error out"=w336:errorcluster, "Done"=w340:bool)  [unwired: 7 in]
              n286 = case shown="True" w340 {
                frame False {
                }
                frame True {
                  n287 = global read "Stage_var.vi" "Stage"() -> (w345:u32)
                  n288 = call <vilib>:"High Resolution Relative Seconds.vi"() -> ("relative seconds"=w343:dbl)
                  n289 = global read "Global_count_var.vi" "Global count"() -> (w341:dbl)
                  n290 = Increment(x=w345) -> (x+1=w344:u32)
                  n291 = global write "Timer.vi" "Timer"(w343) -> ()
                  n292 = global write "Stage_var.vi" "Stage"(w344) -> ()
                  n293 = Increment(x=w341) -> (x+1=w342:dbl)
                  n294 = global write "Global_count_var.vi" "Global count"(w342) -> ()
                }
              }
            }
            frame 24 {
              # "Финишная"
              n295 = call "Forward.vi"("error in (no error)"=w347, "how close"=0.47) -> ("error out"=w346:errorcluster, "Done"=w348:bool)  [unwired: 8 in]
              n296 = case shown="False" w348 {
                frame False {
                }
                frame True {
                  n297 = global read "Stage_var.vi" "Stage"() -> (w354:u32)
                  n298 = global read "Global_count_var.vi" "Global count"() -> (w350:dbl)
                  n299 = call <vilib>:"High Resolution Relative Seconds.vi"() -> ("relative seconds"=w352:dbl)
                  n300 = Increment(x=w354) -> (x+1=w353:u32)
                  n301 = global write "Timer.vi" "Timer"(w352) -> ()
                  n302 = global write "Stage_var.vi" "Stage"(w353) -> ()
                  n303 = Increment(x=w350) -> (x+1=w351:dbl)
                  n304 = global write "Global_count_var.vi" "Global count"(w351) -> ()
                }
              }
            }
            frame 25 {
              # "Поворот на лотки"
              n305 = call "Rotation.vi"("error in (no error)"=w357, "Time"=2.6, "Direction"=-90.0 ("how close")) -> ("error out"=w356:errorcluster, "Done"=w355:bool)  [unwired: 7 in]
              n306 = case shown="True" w355 {
                frame False {
                }
                frame True {
                  n307 = global read "Ball_num_var.vi" "Ball num"() -> (w367:dbl)
                  n308 = call <vilib>:"High Resolution Relative Seconds.vi"() -> ("relative seconds"=w368:dbl)
                  n309 = global write "Stage_var.vi" "Stage"(u32 4 ("Stage")) -> ()
                  n310 = global read "Global_count_var.vi" "Global count"() -> (w360:dbl)
                  n311 = Increment(x=w367) -> (x+1=w366:dbl)
                  n312 = global write "Timer.vi" "Timer"(w368) -> ()
                  n313 = global write "Ball_num_var.vi" "Ball num"(w366) -> ()
                  n314 = Increment(x=w360) -> (x+1=w361:dbl)
                  n315 = global write "Global_count_var.vi" "Global count"(w361) -> ()
                  n316 = global write "Mashina_podyehala.vi" "Mashina podyehala"(FALSE ("Mashina podyehala")) -> ()
                  n317 = global write "Camera_angle.vi" "Camera a"(-0.7 ("Camera a")) -> ()
                  n318 = global write "Arm_stage_var.vi" "Arm stage"(-2.0 ("Arm stage")) -> ()
                }
              }
            }
            frame Default {
            }
          }
        }
        frame 3 {
          n319 = case shown="31" w371 {
            tunnel: w373 -> [w377 w387 w396 w403 w416 w425 w438 w447 w461 w469 w478 w488 w498 w509 w518 w531 w541 w553 w563 w572 w581 w595]
            tunnel: w372 -> [_ _ _ _ _ _ _ _ w460 _ _ _ _ _ _ _ _ _ _ _ _ _]
            tunnel: [w376 w386 w395 w402 w415 w424 w437 w446 w459 w468 w477 w487 w497 w510 w519 w532 w540 w554 w562 w573 w582 w595] -> w370
            frame 13 {
              # "Подъезжаем к перегородке"
              n320 = call "Forward.vi"("error in (no error)"=w377, "how close"=0.5) -> ("error out"=w376:errorcluster, "Done"=w374:bool)  [unwired: 8 in]
              n321 = case shown="True" w374 {
                frame False {
                }
                frame True {
                  n322 = global read "Global_count_var.vi" "Global count"() -> (w378:dbl)
                  n323 = global read "Stage_var.vi" "Stage"() -> (w382:u32)
                  n324 = call <vilib>:"High Resolution Relative Seconds.vi"() -> ("relative seconds"=w380:dbl)
                  n325 = Increment(x=w382) -> (x+1=w381:u32)
                  n326 = global write "Timer.vi" "Timer"(w380) -> ()
                  n327 = global write "Stage_var.vi" "Stage"(w381) -> ()
                  n328 = Increment(x=w378) -> (x+1=w379:dbl)
                  n329 = global write "Global_count_var.vi" "Global count"(w379) -> ()
                }
              }
            }
            frame 14 {
              n330 = call "Rotation.vi"("error in (no error)"=w387, "Time"=2.2, "Direction"=-90.0 ("how close")) -> ("error out"=w386:errorcluster, "Done"=w385:bool)  [unwired: 7 in]
              n331 = case shown="True" w385 {
                frame False {
                }
                frame True {
                  n332 = global read "Stage_var.vi" "Stage"() -> (w392:u32)
                  n333 = call <vilib>:"High Resolution Relative Seconds.vi"() -> ("relative seconds"=w390:dbl)
                  n334 = global read "Global_count_var.vi" "Global count"() -> (w388:dbl)
                  n335 = Increment(x=w392) -> (x+1=w391:u32)
                  n336 = global write "Timer.vi" "Timer"(w390) -> ()
                  n337 = global write "Stage_var.vi" "Stage"(w391) -> ()
                  n338 = Increment(x=w388) -> (x+1=w389:dbl)
                  n339 = global write "Global_count_var.vi" "Global count"(w389) -> ()
                }
              }
            }
            frame 15 {
              n340 = call "Forward_t.vi"("error in (no error)"=w396, "Time"=10.0 ("how close")) -> ("error out"=w395:errorcluster, "Done"=w394:bool)  [unwired: 8 in]
              n341 = case shown="True" w394 {
                frame False {
                }
                frame True {
                  n342 = global read "Global_count_var.vi" "Global count"() -> (w397:dbl)
                  n343 = global read "Stage_var.vi" "Stage"() -> (w401:u32)
                  n344 = call <vilib>:"High Resolution Relative Seconds.vi"() -> ("relative seconds"=w399:dbl)
                  n345 = Increment(x=w401) -> (x+1=w400:u32)
                  n346 = global write "Timer.vi" "Timer"(w399) -> ()
                  n347 = global write "Stage_var.vi" "Stage"(w400) -> ()
                  n348 = Increment(x=w397) -> (x+1=w398:dbl)
                  n349 = global write "Global_count_var.vi" "Global count"(w398) -> ()
                }
              }
            }
            frame 16 {
              # "Поворот к паллету"
              n350 = call "Rotation.vi"("error in (no error)"=w403, "Time"=0.65, "Direction"=-90.0 ("how close")) -> ("error out"=w402:errorcluster, "Done"=w406:bool)  [unwired: 7 in]
              n351 = case shown="True" w406 {
                frame False {
                }
                frame True {
                  n352 = global read "Stage_var.vi" "Stage"() -> (w414:u32)
                  n353 = global read "Global_count_var.vi" "Global count"() -> (w407:dbl)
                  n354 = call <vilib>:"High Resolution Relative Seconds.vi"() -> ("relative seconds"=w412:dbl)
                  n355 = global write "Mashina_podyehala.vi" "Mashina podyehala"(FALSE ("Mashina podyehala")) -> ()
                  n356 = global write "Arm_stage_var.vi" "Arm stage"(-2.0 ("Arm stage")) -> ()
                  n357 = Increment(x=w414) -> (x+1=w413:u32)
                  n358 = global write "Timer.vi" "Timer"(w412) -> ()
                  n359 = global write "Camera_angle.vi" "Camera a"(-0.5 ("Camera a")) -> ()
                  n360 = global write "Stage_var.vi" "Stage"(w413) -> ()
                  n361 = Increment(x=w407) -> (x+1=w408:dbl)
                  n362 = global write "Global_count_var.vi" "Global count"(w408) -> ()
                }
              }
            }
            frame 17 {
              # "Подъезжаем к перегородке"
              n363 = call "Forward.vi"("error in (no error)"=w416, "how close"=0.6) -> ("error out"=w415:errorcluster, "Done"=w417:bool)  [unwired: 8 in]
              n364 = case shown="True" w417 {
                frame False {
                }
                frame True {
                  n365 = global read "Global_count_var.vi" "Global count"() -> (w419:dbl)
                  n366 = global read "Stage_var.vi" "Stage"() -> (w423:u32)
                  n367 = call <vilib>:"High Resolution Relative Seconds.vi"() -> ("relative seconds"=w421:dbl)
                  n368 = Increment(x=w423) -> (x+1=w422:u32)
                  n369 = global write "Timer.vi" "Timer"(w421) -> ()
                  n370 = Increment(x=w419) -> (x+1=w420:dbl)
                  n371 = global write "Stage_var.vi" "Stage"(w422) -> ()
                  n372 = global write "Global_count_var.vi" "Global count"(w420) -> ()
                }
              }
            }
            frame 18 {
              n373 = call "Rotation.vi"("error in (no error)"=w425, "Time"=3.0, "Direction"=-90.0 ("how close")) -> ("error out"=w424:errorcluster, "Done"=w428:bool)  [unwired: 7 in]
              n374 = case shown="True" w428 {
                frame False {
                }
                frame True {
                  n375 = global read "Stage_var.vi" "Stage"() -> (w436:u32)
                  n376 = global read "Global_count_var.vi" "Global count"() -> (w429:dbl)
                  n377 = call <vilib>:"High Resolution Relative Seconds.vi"() -> ("relative seconds"=w434:dbl)
                  n378 = global write "Mashina_podyehala.vi" "Mashina podyehala"(FALSE ("Mashina podyehala")) -> ()
                  n379 = global write "Arm_stage_var.vi" "Arm stage"(-2.0 ("Arm stage")) -> ()
                  n380 = Increment(x=w436) -> (x+1=w435:u32)
                  n381 = global write "Timer.vi" "Timer"(w434) -> ()
                  n382 = global write "Camera_angle.vi" "Camera a"(-0.5 ("Camera a")) -> ()
                  n383 = global write "Stage_var.vi" "Stage"(w435) -> ()
                  n384 = Increment(x=w429) -> (x+1=w430:dbl)
                  n385 = global write "Global_count_var.vi" "Global count"(w430) -> ()
                }
              }
            }
            frame 19 {
              # "Подъезжаем к перегородке"
              n386 = call "Forward.vi"("error in (no error)"=w438, "how close"=0.25) -> ("error out"=w437:errorcluster, "Done"=w439:bool)  [unwired: 8 in]
              n387 = case shown="True" w439 {
                frame False {
                }
                frame True {
                  n388 = global read "Global_count_var.vi" "Global count"() -> (w441:dbl)
                  n389 = global read "Stage_var.vi" "Stage"() -> (w445:u32)
                  n390 = call <vilib>:"High Resolution Relative Seconds.vi"() -> ("relative seconds"=w443:dbl)
                  n391 = Increment(x=w445) -> (x+1=w444:u32)
                  n392 = global write "Timer.vi" "Timer"(w443) -> ()
                  n393 = Increment(x=w441) -> (x+1=w442:dbl)
                  n394 = global write "Stage_var.vi" "Stage"(w444) -> ()
                  n395 = global write "Global_count_var.vi" "Global count"(w442) -> ()
                }
              }
            }
            frame 20 {
              # "Поворот к паллету"
              n396 = call "Rotation.vi"("error in (no error)"=w447, "Time"=3.0, "Direction"=-90.0 ("how close")) -> ("error out"=w446:errorcluster, "Done"=w450:bool)  [unwired: 7 in]
              n397 = case shown="True" w450 {
                frame False {
                }
                frame True {
                  n398 = global read "Stage_var.vi" "Stage"() -> (w458:u32)
                  n399 = global read "Global_count_var.vi" "Global count"() -> (w451:dbl)
                  n400 = call <vilib>:"High Resolution Relative Seconds.vi"() -> ("relative seconds"=w456:dbl)
                  n401 = global write "Mashina_podyehala.vi" "Mashina podyehala"(FALSE ("Mashina podyehala")) -> ()
                  n402 = global write "Arm_stage_var.vi" "Arm stage"(-2.0 ("Arm stage")) -> ()
                  n403 = Increment(x=w458) -> (x+1=w457:u32)
                  n404 = global write "Timer.vi" "Timer"(w456) -> ()
                  n405 = global write "Camera_angle.vi" "Camera a"(-0.5 ("Camera a")) -> ()
                  n406 = global write "Stage_var.vi" "Stage"(w457) -> ()
                  n407 = Increment(x=w451) -> (x+1=w452:dbl)
                  n408 = global write "Global_count_var.vi" "Global count"(w452) -> ()
                }
              }
            }
            frame 21 {
              n409 = call "Put_it.vi"("error in (no error) 2"=w461, "Camera Image"=w460) -> ("error out"=w459:errorcluster, "Done"=w462:bool)  [unwired: 8 in]
              n410 = case shown="True" w462 {
                frame False {
                }
                frame True {
                  n411 = global read "Global_count_var.vi" "Global count"() -> (w463:dbl)
                  n412 = global read "Stage_var.vi" "Stage"() -> (w467:u32)
                  n413 = call <vilib>:"High Resolution Relative Seconds.vi"() -> ("relative seconds"=w465:dbl)
                  n414 = Increment(x=w467) -> (x+1=w466:u32)
                  n415 = global write "Timer.vi" "Timer"(w465) -> ()
                  n416 = Increment(x=w463) -> (x+1=w464:dbl)
                  n417 = global write "Stage_var.vi" "Stage"(w466) -> ()
                  n418 = global write "Global_count_var.vi" "Global count"(w464) -> ()
                }
              }
            }
            frame 22 {
              # "Мы домой едем"
              n419 = call "Backward_t.vi"("error in (no error)"=w469, "Time"=4.0 ("how close")) -> ("error out"=w468:errorcluster, "Done"=w471:bool)  [unwired: 8 in]
              n420 = case shown="False" w471 {
                frame False {
                }
                frame True {
                  n421 = global read "Global_count_var.vi" "Global count"() -> (w472:dbl)
                  n422 = global read "Stage_var.vi" "Stage"() -> (w476:u32)
                  n423 = call <vilib>:"High Resolution Relative Seconds.vi"() -> ("relative seconds"=w474:dbl)
                  n424 = Increment(x=w476) -> (x+1=w475:u32)
                  n425 = global write "Timer.vi" "Timer"(w474) -> ()
                  n426 = Increment(x=w472) -> (x+1=w473:dbl)
                  n427 = global write "Stage_var.vi" "Stage"(w475) -> ()
                  n428 = global write "Global_count_var.vi" "Global count"(w473) -> ()
                }
              }
            }
            frame 23 {
              n429 = call "Rotation.vi"("error in (no error)"=w478, "Time"=2.8, "Direction"=-90.0 ("how close")) -> ("error out"=w477:errorcluster, "Done"=w481:bool)  [unwired: 7 in]
              n430 = case shown="True" w481 {
                frame False {
                }
                frame True {
                  n431 = global read "Stage_var.vi" "Stage"() -> (w486:u32)
                  n432 = call <vilib>:"High Resolution Relative Seconds.vi"() -> ("relative seconds"=w484:dbl)
                  n433 = global read "Global_count_var.vi" "Global count"() -> (w482:dbl)
                  n434 = Increment(x=w486) -> (x+1=w485:u32)
                  n435 = global write "Timer.vi" "Timer"(w484) -> ()
                  n436 = global write "Stage_var.vi" "Stage"(w485) -> ()
                  n437 = Increment(x=w482) -> (x+1=w483:dbl)
                  n438 = global write "Global_count_var.vi" "Global count"(w483) -> ()
                }
              }
            }
            frame 24 {
              n439 = call "Forward.vi"("error in (no error)"=w488, "how close"=0.2) -> ("error out"=w487:errorcluster, "Done"=w489:bool)  [unwired: 8 in]
              n440 = case shown="True" w489 {
                frame False {
                }
                frame True {
                  n441 = global read "Stage_var.vi" "Stage"() -> (w495:u32)
                  n442 = global read "Global_count_var.vi" "Global count"() -> (w491:dbl)
                  n443 = call <vilib>:"High Resolution Relative Seconds.vi"() -> ("relative seconds"=w493:dbl)
                  n444 = Increment(x=w495) -> (x+1=w494:u32)
                  n445 = global write "Timer.vi" "Timer"(w493) -> ()
                  n446 = global write "Stage_var.vi" "Stage"(w494) -> ()
                  n447 = Increment(x=w491) -> (x+1=w492:dbl)
                  n448 = global write "Global_count_var.vi" "Global count"(w492) -> ()
                }
              }
            }
            frame 25 {
              n449 = call "Rotation.vi"("error in (no error)"=w498, "Time"=3.0, "Direction"=90.0 ("how close")) -> ("error out"=w497:errorcluster, "Done"=w496:bool)  [unwired: 7 in]
              n450 = case shown="True" w496 {
                frame False {
                }
                frame True {
                  n451 = global read "Stage_var.vi" "Stage"() -> (w503:u32)
                  n452 = call <vilib>:"High Resolution Relative Seconds.vi"() -> ("relative seconds"=w508:dbl)
                  n453 = global read "Global_count_var.vi" "Global count"() -> (w501:dbl)
                  n454 = Increment(x=w503) -> (x+1=w504:u32)
                  n455 = global write "Timer.vi" "Timer"(w508) -> ()
                  n456 = global write "Stage_var.vi" "Stage"(w504) -> ()
                  n457 = Increment(x=w501) -> (x+1=w502:dbl)
                  n458 = global write "Global_count_var.vi" "Global count"(w502) -> ()
                  n459 = global write "Mashina_podyehala.vi" "Mashina podyehala"(FALSE ("Mashina podyehala")) -> ()
                  n460 = global write "Camera_angle.vi" "Camera a"(-0.7 ("Camera a")) -> ()
                  n461 = global write "Arm_stage_var.vi" "Arm stage"(-2.0 ("Arm stage")) -> ()
                }
              }
            }
            frame 26 {
              n462 = call "Forward_t.vi"("error in (no error)"=w509, "Time"=4.0 ("how close")) -> ("error out"=w510:errorcluster, "Done"=w512:bool)  [unwired: 8 in]
              n463 = case shown="True" w512 {
                frame False {
                }
                frame True {
                  n464 = global read "Stage_var.vi" "Stage"() -> (w517:u32)
                  n465 = global read "Global_count_var.vi" "Global count"() -> (w513:dbl)
                  n466 = call <vilib>:"High Resolution Relative Seconds.vi"() -> ("relative seconds"=w515:dbl)
                  n467 = Increment(x=w517) -> (x+1=w516:u32)
                  n468 = global write "Timer.vi" "Timer"(w515) -> ()
                  n469 = global write "Stage_var.vi" "Stage"(w516) -> ()
                  n470 = Increment(x=w513) -> (x+1=w514:dbl)
                  n471 = global write "Global_count_var.vi" "Global count"(w514) -> ()
                }
              }
            }
            frame 27 {
              n472 = call "Rotation.vi"("error in (no error)"=w518, "Time"=1.0, "Direction"=90.0 ("how close")) -> ("error out"=w519:errorcluster, "Done"=w520:bool)  [unwired: 7 in]
              n473 = case shown="True" w520 {
                frame False {
                }
                frame True {
                  n474 = global read "Stage_var.vi" "Stage"() -> (w526:u32)
                  n475 = call <vilib>:"High Resolution Relative Seconds.vi"() -> ("relative seconds"=w530:dbl)
                  n476 = global read "Global_count_var.vi" "Global count"() -> (w523:dbl)
                  n477 = Increment(x=w526) -> (x+1=w525:u32)
                  n478 = global write "Timer.vi" "Timer"(w530) -> ()
                  n479 = global write "Stage_var.vi" "Stage"(w525) -> ()
                  n480 = Increment(x=w523) -> (x+1=w524:dbl)
                  n481 = global write "Global_count_var.vi" "Global count"(w524) -> ()
                  n482 = global write "Mashina_podyehala.vi" "Mashina podyehala"(FALSE ("Mashina podyehala")) -> ()
                  n483 = global write "Camera_angle.vi" "Camera a"(-0.7 ("Camera a")) -> ()
                  n484 = global write "Arm_stage_var.vi" "Arm stage"(-2.0 ("Arm stage")) -> ()
                }
              }
            }
            frame 28 {
              n485 = call "Forward_t.vi"("error in (no error)"=w531, "Time"=11.0 ("how close")) -> ("error out"=w532:errorcluster, "Done"=w534:bool)  [unwired: 8 in]
              n486 = case shown="True" w534 {
                frame False {
                }
                frame True {
                  n487 = global read "Stage_var.vi" "Stage"() -> (w539:u32)
                  n488 = call <vilib>:"High Resolution Relative Seconds.vi"() -> ("relative seconds"=w537:dbl)
                  n489 = global read "Global_count_var.vi" "Global count"() -> (w535:dbl)
                  n490 = Increment(x=w539) -> (x+1=w538:u32)
                  n491 = global write "Timer.vi" "Timer"(w537) -> ()
                  n492 = global write "Stage_var.vi" "Stage"(w538) -> ()
                  n493 = Increment(x=w535) -> (x+1=w536:dbl)
                  n494 = global write "Global_count_var.vi" "Global count"(w536) -> ()
                }
              }
            }
            frame 29 {
              n495 = call "Rotation.vi"("error in (no error)"=w541, "Time"=2.0, "Direction"=90.0 ("how close")) -> ("error out"=w540:errorcluster, "Done"=w542:bool)  [unwired: 7 in]
              n496 = case shown="False" w542 {
                frame False {
                }
                frame True {
                  n497 = global read "Stage_var.vi" "Stage"() -> (w548:u32)
                  n498 = call <vilib>:"High Resolution Relative Seconds.vi"() -> ("relative seconds"=w552:dbl)
                  n499 = global read "Global_count_var.vi" "Global count"() -> (w545:dbl)
                  n500 = Increment(x=w548) -> (x+1=w547:u32)
                  n501 = global write "Timer.vi" "Timer"(w552) -> ()
                  n502 = global write "Stage_var.vi" "Stage"(w547) -> ()
                  n503 = Increment(x=w545) -> (x+1=w546:dbl)
                  n504 = global write "Global_count_var.vi" "Global count"(w546) -> ()
                  n505 = global write "Mashina_podyehala.vi" "Mashina podyehala"(FALSE ("Mashina podyehala")) -> ()
                  n506 = global write "Camera_angle.vi" "Camera a"(-0.7 ("Camera a")) -> ()
                  n507 = global write "Arm_stage_var.vi" "Arm stage"(-2.0 ("Arm stage")) -> ()
                }
              }
            }
            frame 30 {
              n508 = call "Forward.vi"("error in (no error)"=w553, "how close"=0.17) -> ("error out"=w554:errorcluster, "Done"=w555:bool)  [unwired: 8 in]
              n509 = case shown="True" w555 {
                frame False {
                }
                frame True {
                  n510 = global read "Stage_var.vi" "Stage"() -> (w561:u32)
                  n511 = call <vilib>:"High Resolution Relative Seconds.vi"() -> ("relative seconds"=w559:dbl)
                  n512 = global read "Global_count_var.vi" "Global count"() -> (w557:dbl)
                  n513 = Increment(x=w561) -> (x+1=w560:u32)
                  n514 = global write "Timer.vi" "Timer"(w559) -> ()
                  n515 = global write "Stage_var.vi" "Stage"(w560) -> ()
                  n516 = Increment(x=w557) -> (x+1=w558:dbl)
                  n517 = global write "Global_count_var.vi" "Global count"(w558) -> ()
                }
              }
            }
            frame 31 {
              # "B"
              n518 = call "Rotation.vi"("error in (no error)"=w563, "Time"=2.8, "Direction"=-90.0 ("how close")) -> ("error out"=w562:errorcluster, "Done"=w566:bool)  [unwired: 7 in]
              n519 = case shown="True" w566 {
                frame False {
                }
                frame True {
                  n520 = global read "Stage_var.vi" "Stage"() -> (w571:u32)
                  n521 = call <vilib>:"High Resolution Relative Seconds.vi"() -> ("relative seconds"=w569:dbl)
                  n522 = global read "Global_count_var.vi" "Global count"() -> (w567:dbl)
                  n523 = Increment(x=w571) -> (x+1=w570:u32)
                  n524 = global write "Timer.vi" "Timer"(w569) -> ()
                  n525 = global write "Stage_var.vi" "Stage"(w570) -> ()
                  n526 = Increment(x=w567) -> (x+1=w568:dbl)
                  n527 = global write "Global_count_var.vi" "Global count"(w568) -> ()
                }
              }
            }
            frame 32 {
              # "Финишная"
              n528 = call "Forward.vi"("error in (no error)"=w572, "how close"=0.47) -> ("error out"=w573:errorcluster, "Done"=w574:bool)  [unwired: 8 in]
              n529 = case shown="True" w574 {
                frame False {
                }
                frame True {
                  n530 = global read "Stage_var.vi" "Stage"() -> (w580:u32)
                  n531 = global read "Global_count_var.vi" "Global count"() -> (w576:dbl)
                  n532 = call <vilib>:"High Resolution Relative Seconds.vi"() -> ("relative seconds"=w578:dbl)
                  n533 = Increment(x=w580) -> (x+1=w579:u32)
                  n534 = global write "Timer.vi" "Timer"(w578) -> ()
                  n535 = global write "Stage_var.vi" "Stage"(w579) -> ()
                  n536 = Increment(x=w576) -> (x+1=w577:dbl)
                  n537 = global write "Global_count_var.vi" "Global count"(w577) -> ()
                }
              }
            }
            frame 33 {
              # "Поворот на лотки"
              n538 = call "Rotation.vi"("error in (no error)"=w581, "Time"=2.6, "Direction"=-90.0 ("how close")) -> ("error out"=w582:errorcluster, "Done"=w583:bool)  [unwired: 7 in]
              n539 = case shown="True" w583 {
                frame False {
                }
                frame True {
                  n540 = global read "Ball_num_var.vi" "Ball num"() -> (w593:dbl)
                  n541 = call <vilib>:"High Resolution Relative Seconds.vi"() -> ("relative seconds"=w594:dbl)
                  n542 = global read "Global_count_var.vi" "Global count"() -> (w586:dbl)
                  n543 = global write "Stage_var.vi" "Stage"(u32 4 ("Stage")) -> ()
                  n544 = Increment(x=w593) -> (x+1=w592:dbl)
                  n545 = global write "Timer.vi" "Timer"(w594) -> ()
                  n546 = global write "Ball_num_var.vi" "Ball num"(w592) -> ()
                  n547 = Increment(x=w586) -> (x+1=w587:dbl)
                  n548 = global write "Global_count_var.vi" "Global count"(w587) -> ()
                  n549 = global write "Mashina_podyehala.vi" "Mashina podyehala"(FALSE ("Mashina podyehala")) -> ()
                  n550 = global write "Camera_angle.vi" "Camera a"(-0.7 ("Camera a")) -> ()
                  n551 = global write "Arm_stage_var.vi" "Arm stage"(-2.0 ("Arm stage")) -> ()
                }
              }
            }
            frame Default {
            }
          }
        }
        frame 4 {
          n552 = case shown="31" w599 {
            tunnel: w598 -> [w603 w613 w622 w629 w642 w651 w664 w673 w687 w695 w704 w714 w724 w735 w744 w757 w767 w779 w789 w798 w807 w821]
            tunnel: w597 -> [_ _ _ _ _ _ _ _ w686 _ _ _ _ _ _ _ _ _ _ _ _ _]
            tunnel: [w602 w612 w621 w628 w641 w650 w663 w672 w685 w694 w703 w713 w723 w736 w745 w758 w766 w780 w788 w799 w808 w821] -> w596
            frame 13 {
              # "Подъезжаем к перегородке"
              n553 = call "Forward.vi"("error in (no error)"=w603, "how close"=0.5) -> ("error out"=w602:errorcluster, "Done"=w600:bool)  [unwired: 8 in]
              n554 = case shown="True" w600 {
                frame False {
                }
                frame True {
                  n555 = global read "Stage_var.vi" "Stage"() -> (w608:u32)
                  n556 = global read "Global_count_var.vi" "Global count"() -> (w604:dbl)
                  n557 = call <vilib>:"High Resolution Relative Seconds.vi"() -> ("relative seconds"=w606:dbl)
                  n558 = Increment(x=w608) -> (x+1=w607:u32)
                  n559 = global write "Timer.vi" "Timer"(w606) -> ()
                  n560 = global write "Stage_var.vi" "Stage"(w607) -> ()
                  n561 = Increment(x=w604) -> (x+1=w605:dbl)
                  n562 = global write "Global_count_var.vi" "Global count"(w605) -> ()
                }
              }
            }
            frame 14 {
              n563 = call "Rotation.vi"("error in (no error)"=w613, "Time"=2.2, "Direction"=-90.0 ("how close")) -> ("error out"=w612:errorcluster, "Done"=w611:bool)  [unwired: 7 in]
              n564 = case shown="True" w611 {
                frame False {
                }
                frame True {
                  n565 = global read "Stage_var.vi" "Stage"() -> (w618:u32)
                  n566 = call <vilib>:"High Resolution Relative Seconds.vi"() -> ("relative seconds"=w616:dbl)
                  n567 = global read "Global_count_var.vi" "Global count"() -> (w614:dbl)
                  n568 = Increment(x=w618) -> (x+1=w617:u32)
                  n569 = global write "Timer.vi" "Timer"(w616) -> ()
                  n570 = global write "Stage_var.vi" "Stage"(w617) -> ()
                  n571 = Increment(x=w614) -> (x+1=w615:dbl)
                  n572 = global write "Global_count_var.vi" "Global count"(w615) -> ()
                }
              }
            }
            frame 15 {
              n573 = call "Forward_t.vi"("error in (no error)"=w622, "Time"=10.0 ("how close")) -> ("error out"=w621:errorcluster, "Done"=w620:bool)  [unwired: 8 in]
              n574 = case shown="True" w620 {
                frame False {
                }
                frame True {
                  n575 = global read "Stage_var.vi" "Stage"() -> (w627:u32)
                  n576 = global read "Global_count_var.vi" "Global count"() -> (w623:dbl)
                  n577 = call <vilib>:"High Resolution Relative Seconds.vi"() -> ("relative seconds"=w625:dbl)
                  n578 = Increment(x=w627) -> (x+1=w626:u32)
                  n579 = global write "Timer.vi" "Timer"(w625) -> ()
                  n580 = global write "Stage_var.vi" "Stage"(w626) -> ()
                  n581 = Increment(x=w623) -> (x+1=w624:dbl)
                  n582 = global write "Global_count_var.vi" "Global count"(w624) -> ()
                }
              }
            }
            frame 16 {
              # "Поворот к паллету"
              n583 = call "Rotation.vi"("error in (no error)"=w629, "Time"=0.65, "Direction"=-90.0 ("how close")) -> ("error out"=w628:errorcluster, "Done"=w632:bool)  [unwired: 7 in]
              n584 = case shown="True" w632 {
                frame False {
                }
                frame True {
                  n585 = global read "Stage_var.vi" "Stage"() -> (w640:u32)
                  n586 = call <vilib>:"High Resolution Relative Seconds.vi"() -> ("relative seconds"=w638:dbl)
                  n587 = global write "Mashina_podyehala.vi" "Mashina podyehala"(FALSE ("Mashina podyehala")) -> ()
                  n588 = global read "Global_count_var.vi" "Global count"() -> (w633:dbl)
                  n589 = global write "Arm_stage_var.vi" "Arm stage"(-1.0 ("Arm stage")) -> ()
                  n590 = Increment(x=w640) -> (x+1=w639:u32)
                  n591 = global write "Timer.vi" "Timer"(w638) -> ()
                  n592 = global write "Camera_angle.vi" "Camera a"(-0.5 ("Camera a")) -> ()
                  n593 = global write "Stage_var.vi" "Stage"(w639) -> ()
                  n594 = Increment(x=w633) -> (x+1=w634:dbl)
                  n595 = global write "Global_count_var.vi" "Global count"(w634) -> ()
                }
              }
            }
            frame 17 {
              # "Подъезжаем к перегородке"
              n596 = call "Forward.vi"("error in (no error)"=w642, "how close"=0.6) -> ("error out"=w641:errorcluster, "Done"=w643:bool)  [unwired: 8 in]
              n597 = case shown="True" w643 {
                frame False {
                }
                frame True {
                  n598 = global read "Global_count_var.vi" "Global count"() -> (w645:dbl)
                  n599 = global read "Stage_var.vi" "Stage"() -> (w649:u32)
                  n600 = call <vilib>:"High Resolution Relative Seconds.vi"() -> ("relative seconds"=w647:dbl)
                  n601 = Increment(x=w649) -> (x+1=w648:u32)
                  n602 = global write "Timer.vi" "Timer"(w647) -> ()
                  n603 = global write "Stage_var.vi" "Stage"(w648) -> ()
                  n604 = Increment(x=w645) -> (x+1=w646:dbl)
                  n605 = global write "Global_count_var.vi" "Global count"(w646) -> ()
                }
              }
            }
            frame 18 {
              # "Поворот к паллету"
              n606 = call "Rotation.vi"("error in (no error)"=w651, "Time"=3.0, "Direction"=-90.0 ("how close")) -> ("error out"=w650:errorcluster, "Done"=w654:bool)  [unwired: 7 in]
              n607 = case shown="True" w654 {
                frame False {
                }
                frame True {
                  n608 = global read "Stage_var.vi" "Stage"() -> (w662:u32)
                  n609 = call <vilib>:"High Resolution Relative Seconds.vi"() -> ("relative seconds"=w660:dbl)
                  n610 = global write "Mashina_podyehala.vi" "Mashina podyehala"(FALSE ("Mashina podyehala")) -> ()
                  n611 = global write "Arm_stage_var.vi" "Arm stage"(-1.0 ("Arm stage")) -> ()
                  n612 = global read "Global_count_var.vi" "Global count"() -> (w655:dbl)
                  n613 = Increment(x=w662) -> (x+1=w661:u32)
                  n614 = global write "Timer.vi" "Timer"(w660) -> ()
                  n615 = global write "Camera_angle.vi" "Camera a"(-0.5 ("Camera a")) -> ()
                  n616 = global write "Stage_var.vi" "Stage"(w661) -> ()
                  n617 = Increment(x=w655) -> (x+1=w656:dbl)
                  n618 = global write "Global_count_var.vi" "Global count"(w656) -> ()
                }
              }
            }
            frame 19 {
              # "Подъезжаем к перегородке"
              n619 = call "Forward.vi"("error in (no error)"=w664, "how close"=0.25) -> ("error out"=w663:errorcluster, "Done"=w665:bool)  [unwired: 8 in]
              n620 = case shown="True" w665 {
                frame False {
                }
                frame True {
                  n621 = global read "Global_count_var.vi" "Global count"() -> (w667:dbl)
                  n622 = global read "Stage_var.vi" "Stage"() -> (w671:u32)
                  n623 = call <vilib>:"High Resolution Relative Seconds.vi"() -> ("relative seconds"=w669:dbl)
                  n624 = Increment(x=w671) -> (x+1=w670:u32)
                  n625 = global write "Timer.vi" "Timer"(w669) -> ()
                  n626 = global write "Stage_var.vi" "Stage"(w670) -> ()
                  n627 = Increment(x=w667) -> (x+1=w668:dbl)
                  n628 = global write "Global_count_var.vi" "Global count"(w668) -> ()
                }
              }
            }
            frame 20 {
              # "Поворот к паллету"
              n629 = call "Rotation.vi"("error in (no error)"=w673, "Time"=3.0, "Direction"=90.0 ("how close")) -> ("error out"=w672:errorcluster, "Done"=w676:bool)  [unwired: 7 in]
              n630 = case shown="True" w676 {
                frame False {
                }
                frame True {
                  n631 = global read "Stage_var.vi" "Stage"() -> (w684:u32)
                  n632 = call <vilib>:"High Resolution Relative Seconds.vi"() -> ("relative seconds"=w682:dbl)
                  n633 = global read "Global_count_var.vi" "Global count"() -> (w677:dbl)
                  n634 = global write "Mashina_podyehala.vi" "Mashina podyehala"(FALSE ("Mashina podyehala")) -> ()
                  n635 = global write "Arm_stage_var.vi" "Arm stage"(-2.0 ("Arm stage")) -> ()
                  n636 = Increment(x=w684) -> (x+1=w683:u32)
                  n637 = global write "Timer.vi" "Timer"(w682) -> ()
                  n638 = global write "Camera_angle.vi" "Camera a"(-0.5 ("Camera a")) -> ()
                  n639 = global write "Stage_var.vi" "Stage"(w683) -> ()
                  n640 = Increment(x=w677) -> (x+1=w678:dbl)
                  n641 = global write "Global_count_var.vi" "Global count"(w678) -> ()
                }
              }
            }
            frame 21 {
              n642 = call "Put_it.vi"("error in (no error) 2"=w687, "Camera Image"=w686) -> ("error out"=w685:errorcluster, "Done"=w688:bool)  [unwired: 8 in]
              n643 = case shown="False" w688 {
                frame False {
                }
                frame True {
                  n644 = global read "Global_count_var.vi" "Global count"() -> (w689:dbl)
                  n645 = global read "Stage_var.vi" "Stage"() -> (w693:u32)
                  n646 = call <vilib>:"High Resolution Relative Seconds.vi"() -> ("relative seconds"=w691:dbl)
                  n647 = Increment(x=w693) -> (x+1=w692:u32)
                  n648 = global write "Timer.vi" "Timer"(w691) -> ()
                  n649 = global write "Stage_var.vi" "Stage"(w692) -> ()
                  n650 = Increment(x=w689) -> (x+1=w690:dbl)
                  n651 = global write "Global_count_var.vi" "Global count"(w690) -> ()
                }
              }
            }
            frame 22 {
              # "Мы домой едем"
              n652 = call "Backward_t.vi"("error in (no error)"=w695, "Time"=4.0 ("how close")) -> ("error out"=w694:errorcluster, "Done"=w697:bool)  [unwired: 8 in]
              n653 = case shown="True" w697 {
                frame False {
                }
                frame True {
                  n654 = global read "Global_count_var.vi" "Global count"() -> (w698:dbl)
                  n655 = global read "Stage_var.vi" "Stage"() -> (w702:u32)
                  n656 = call <vilib>:"High Resolution Relative Seconds.vi"() -> ("relative seconds"=w700:dbl)
                  n657 = Increment(x=w702) -> (x+1=w701:u32)
                  n658 = global write "Timer.vi" "Timer"(w700) -> ()
                  n659 = global write "Stage_var.vi" "Stage"(w701) -> ()
                  n660 = Increment(x=w698) -> (x+1=w699:dbl)
                  n661 = global write "Global_count_var.vi" "Global count"(w699) -> ()
                }
              }
            }
            frame 23 {
              # "Y"
              n662 = call "Rotation.vi"("error in (no error)"=w704, "Time"=2.8, "Direction"=90.0 ("how close")) -> ("error out"=w703:errorcluster, "Done"=w707:bool)  [unwired: 7 in]
              n663 = case shown="True" w707 {
                frame False {
                }
                frame True {
                  n664 = global read "Stage_var.vi" "Stage"() -> (w712:u32)
                  n665 = call <vilib>:"High Resolution Relative Seconds.vi"() -> ("relative seconds"=w710:dbl)
                  n666 = global read "Global_count_var.vi" "Global count"() -> (w708:dbl)
                  n667 = Increment(x=w712) -> (x+1=w711:u32)
                  n668 = global write "Timer.vi" "Timer"(w710) -> ()
                  n669 = global write "Stage_var.vi" "Stage"(w711) -> ()
                  n670 = Increment(x=w708) -> (x+1=w709:dbl)
                  n671 = global write "Global_count_var.vi" "Global count"(w709) -> ()
                }
              }
            }
            frame 24 {
              n672 = call "Forward.vi"("error in (no error)"=w714, "how close"=0.2) -> ("error out"=w713:errorcluster, "Done"=w715:bool)  [unwired: 8 in]
              n673 = case shown="True" w715 {
                frame False {
                }
                frame True {
                  n674 = global read "Stage_var.vi" "Stage"() -> (w721:u32)
                  n675 = call <vilib>:"High Resolution Relative Seconds.vi"() -> ("relative seconds"=w719:dbl)
                  n676 = global read "Global_count_var.vi" "Global count"() -> (w717:dbl)
                  n677 = Increment(x=w721) -> (x+1=w720:u32)
                  n678 = global write "Timer.vi" "Timer"(w719) -> ()
                  n679 = global write "Stage_var.vi" "Stage"(w720) -> ()
                  n680 = Increment(x=w717) -> (x+1=w718:dbl)
                  n681 = global write "Global_count_var.vi" "Global count"(w718) -> ()
                }
              }
            }
            frame 25 {
              n682 = call "Rotation.vi"("error in (no error)"=w724, "Time"=3.0, "Direction"=90.0 ("how close")) -> ("error out"=w723:errorcluster, "Done"=w722:bool)  [unwired: 7 in]
              n683 = case shown="True" w722 {
                frame False {
                }
                frame True {
                  n684 = global read "Stage_var.vi" "Stage"() -> (w729:u32)
                  n685 = call <vilib>:"High Resolution Relative Seconds.vi"() -> ("relative seconds"=w734:dbl)
                  n686 = global read "Global_count_var.vi" "Global count"() -> (w727:dbl)
                  n687 = Increment(x=w729) -> (x+1=w730:u32)
                  n688 = global write "Timer.vi" "Timer"(w734) -> ()
                  n689 = global write "Stage_var.vi" "Stage"(w730) -> ()
                  n690 = Increment(x=w727) -> (x+1=w728:dbl)
                  n691 = global write "Mashina_podyehala.vi" "Mashina podyehala"(FALSE ("Mashina podyehala")) -> ()
                  n692 = global write "Global_count_var.vi" "Global count"(w728) -> ()
                  n693 = global write "Camera_angle.vi" "Camera a"(-0.7 ("Camera a")) -> ()
                  n694 = global write "Arm_stage_var.vi" "Arm stage"(-2.0 ("Arm stage")) -> ()
                }
              }
            }
            frame 26 {
              n695 = call "Forward_t.vi"("error in (no error)"=w735, "Time"=4.0 ("how close")) -> ("error out"=w736:errorcluster, "Done"=w738:bool)  [unwired: 8 in]
              n696 = case shown="True" w738 {
                frame False {
                }
                frame True {
                  n697 = global read "Stage_var.vi" "Stage"() -> (w743:u32)
                  n698 = call <vilib>:"High Resolution Relative Seconds.vi"() -> ("relative seconds"=w741:dbl)
                  n699 = global read "Global_count_var.vi" "Global count"() -> (w739:dbl)
                  n700 = Increment(x=w743) -> (x+1=w742:u32)
                  n701 = global write "Timer.vi" "Timer"(w741) -> ()
                  n702 = global write "Stage_var.vi" "Stage"(w742) -> ()
                  n703 = Increment(x=w739) -> (x+1=w740:dbl)
                  n704 = global write "Global_count_var.vi" "Global count"(w740) -> ()
                }
              }
            }
            frame 27 {
              n705 = call "Rotation.vi"("error in (no error)"=w744, "Time"=1.0, "Direction"=90.0 ("how close")) -> ("error out"=w745:errorcluster, "Done"=w746:bool)  [unwired: 7 in]
              n706 = case shown="True" w746 {
                frame False {
                }
                frame True {
                  n707 = global read "Stage_var.vi" "Stage"() -> (w752:u32)
                  n708 = call <vilib>:"High Resolution Relative Seconds.vi"() -> ("relative seconds"=w756:dbl)
                  n709 = global read "Global_count_var.vi" "Global count"() -> (w749:dbl)
                  n710 = Increment(x=w752) -> (x+1=w751:u32)
                  n711 = global write "Timer.vi" "Timer"(w756) -> ()
                  n712 = global write "Stage_var.vi" "Stage"(w751) -> ()
                  n713 = Increment(x=w749) -> (x+1=w750:dbl)
                  n714 = global write "Global_count_var.vi" "Global count"(w750) -> ()
                  n715 = global write "Mashina_podyehala.vi" "Mashina podyehala"(FALSE ("Mashina podyehala")) -> ()
                  n716 = global write "Camera_angle.vi" "Camera a"(-0.7 ("Camera a")) -> ()
                  n717 = global write "Arm_stage_var.vi" "Arm stage"(-1.0 ("Arm stage")) -> ()
                }
              }
            }
            frame 28 {
              n718 = call "Forward_t.vi"("error in (no error)"=w757, "Time"=11.0 ("how close")) -> ("error out"=w758:errorcluster, "Done"=w760:bool)  [unwired: 8 in]
              n719 = case shown="True" w760 {
                frame False {
                }
                frame True {
                  n720 = global read "Stage_var.vi" "Stage"() -> (w765:u32)
                  n721 = call <vilib>:"High Resolution Relative Seconds.vi"() -> ("relative seconds"=w763:dbl)
                  n722 = global read "Global_count_var.vi" "Global count"() -> (w761:dbl)
                  n723 = Increment(x=w765) -> (x+1=w764:u32)
                  n724 = global write "Timer.vi" "Timer"(w763) -> ()
                  n725 = global write "Stage_var.vi" "Stage"(w764) -> ()
                  n726 = Increment(x=w761) -> (x+1=w762:dbl)
                  n727 = global write "Global_count_var.vi" "Global count"(w762) -> ()
                }
              }
            }
            frame 29 {
              n728 = call "Rotation.vi"("error in (no error)"=w767, "Time"=2.0, "Direction"=90.0 ("how close")) -> ("error out"=w766:errorcluster, "Done"=w768:bool)  [unwired: 7 in]
              n729 = case shown="True" w768 {
                frame False {
                }
                frame True {
                  n730 = global read "Stage_var.vi" "Stage"() -> (w774:u32)
                  n731 = call <vilib>:"High Resolution Relative Seconds.vi"() -> ("relative seconds"=w778:dbl)
                  n732 = global read "Global_count_var.vi" "Global count"() -> (w771:dbl)
                  n733 = Increment(x=w774) -> (x+1=w773:u32)
                  n734 = global write "Timer.vi" "Timer"(w778) -> ()
                  n735 = global write "Stage_var.vi" "Stage"(w773) -> ()
                  n736 = Increment(x=w771) -> (x+1=w772:dbl)
                  n737 = global write "Global_count_var.vi" "Global count"(w772) -> ()
                  n738 = global write "Mashina_podyehala.vi" "Mashina podyehala"(FALSE ("Mashina podyehala")) -> ()
                  n739 = global write "Camera_angle.vi" "Camera a"(-0.7 ("Camera a")) -> ()
                  n740 = global write "Arm_stage_var.vi" "Arm stage"(-2.0 ("Arm stage")) -> ()
                }
              }
            }
            frame 30 {
              n741 = call "Forward.vi"("error in (no error)"=w779, "how close"=0.18) -> ("error out"=w780:errorcluster, "Done"=w781:bool)  [unwired: 8 in]
              n742 = case shown="True" w781 {
                frame False {
                }
                frame True {
                  n743 = global read "Stage_var.vi" "Stage"() -> (w787:u32)
                  n744 = call <vilib>:"High Resolution Relative Seconds.vi"() -> ("relative seconds"=w785:dbl)
                  n745 = global read "Global_count_var.vi" "Global count"() -> (w783:dbl)
                  n746 = Increment(x=w787) -> (x+1=w786:u32)
                  n747 = global write "Timer.vi" "Timer"(w785) -> ()
                  n748 = global write "Stage_var.vi" "Stage"(w786) -> ()
                  n749 = Increment(x=w783) -> (x+1=w784:dbl)
                  n750 = global write "Global_count_var.vi" "Global count"(w784) -> ()
                }
              }
            }
            frame 31 {
              n751 = call "Rotation.vi"("error in (no error)"=w789, "Time"=2.8, "Direction"=-90.0 ("how close")) -> ("error out"=w788:errorcluster, "Done"=w792:bool)  [unwired: 7 in]
              n752 = case shown="True" w792 {
                frame False {
                }
                frame True {
                  n753 = global read "Stage_var.vi" "Stage"() -> (w797:u32)
                  n754 = call <vilib>:"High Resolution Relative Seconds.vi"() -> ("relative seconds"=w795:dbl)
                  n755 = Increment(x=w797) -> (x+1=w796:u32)
                  n756 = global read "Global_count_var.vi" "Global count"() -> (w793:dbl)
                  n757 = global write "Timer.vi" "Timer"(w795) -> ()
                  n758 = global write "Stage_var.vi" "Stage"(w796) -> ()
                  n759 = Increment(x=w793) -> (x+1=w794:dbl)
                  n760 = global write "Global_count_var.vi" "Global count"(w794) -> ()
                }
              }
            }
            frame 32 {
              # "Финишная"
              n761 = call "Forward.vi"("error in (no error)"=w798, "how close"=0.47) -> ("error out"=w799:errorcluster, "Done"=w800:bool)  [unwired: 8 in]
              n762 = case shown="True" w800 {
                frame False {
                }
                frame True {
                  n763 = global read "Stage_var.vi" "Stage"() -> (w806:u32)
                  n764 = global read "Global_count_var.vi" "Global count"() -> (w802:dbl)
                  n765 = call <vilib>:"High Resolution Relative Seconds.vi"() -> ("relative seconds"=w804:dbl)
                  n766 = Increment(x=w806) -> (x+1=w805:u32)
                  n767 = global write "Timer.vi" "Timer"(w804) -> ()
                  n768 = global write "Stage_var.vi" "Stage"(w805) -> ()
                  n769 = Increment(x=w802) -> (x+1=w803:dbl)
                  n770 = global write "Global_count_var.vi" "Global count"(w803) -> ()
                }
              }
            }
            frame 33 {
              # "Поворот на лотки"
              n771 = call "Rotation.vi"("error in (no error)"=w807, "Time"=2.6, "Direction"=-90.0 ("how close")) -> ("error out"=w808:errorcluster, "Done"=w809:bool)  [unwired: 7 in]
              n772 = case shown="True" w809 {
                frame False {
                }
                frame True {
                  n773 = global read "Ball_num_var.vi" "Ball num"() -> (w819:dbl)
                  n774 = call <vilib>:"High Resolution Relative Seconds.vi"() -> ("relative seconds"=w820:dbl)
                  n775 = global write "Stage_var.vi" "Stage"(u32 4 ("Stage")) -> ()
                  n776 = Increment(x=w819) -> (x+1=w818:dbl)
                  n777 = global write "Timer.vi" "Timer"(w820) -> ()
                  n778 = global read "Global_count_var.vi" "Global count"() -> (w812:dbl)
                  n779 = global write "Ball_num_var.vi" "Ball num"(w818) -> ()
                  n780 = Increment(x=w812) -> (x+1=w813:dbl)
                  n781 = global write "Mashina_podyehala.vi" "Mashina podyehala"(FALSE ("Mashina podyehala")) -> ()
                  n782 = global write "Camera_angle.vi" "Camera a"(-0.7 ("Camera a")) -> ()
                  n783 = global write "Global_count_var.vi" "Global count"(w813) -> ()
                  n784 = global write "Arm_stage_var.vi" "Arm stage"(-2.0 ("Arm stage")) -> ()
                }
              }
            }
            frame Default {
            }
          }
        }
      }
      n785 = case shown="4" w90 {
        tunnel: w88 -> [w824 w865 w896 w924 w946 w968 w977 w986 w996 w1005]
        tunnel: [w823 w864 w908 w925 w945 w967 w976 w987 w995 w1005] -> w96
        tunnel: w91 -> [_ _ w893 _ _ _ _ _ _ _]
        frame 4 {
          n786 = global read "Ball_num_var.vi" "Ball num"() -> (w822:dbl)
          n787 = case shown="4" w822 {
            tunnel: w824 -> [w826 w834 w843 w853 w857]
            tunnel: [w825 w835 w844 w853 w856] -> w823
            frame 2 {
              n788 = call "Forward.vi"("error in (no error)"=w826, "how close"=0.3) -> ("error out"=w825:errorcluster, "Done"=w827:bool)  [unwired: 8 in]
              n789 = case shown="True" w827 {
                frame False {
                }
                frame True {
                  n790 = global read "Stage_var.vi" "Stage"() -> (w833:u32)
                  n791 = call <vilib>:"High Resolution Relative Seconds.vi"() -> ("relative seconds"=w831:dbl)
                  n792 = global read "Global_count_var.vi" "Global count"() -> (w829:dbl)
                  n793 = Increment(x=w833) -> (x+1=w832:u32)
                  n794 = global write "Timer.vi" "Timer"(w831) -> ()
                  n795 = global write "Stage_var.vi" "Stage"(w832) -> ()
                  n796 = Increment(x=w829) -> (x+1=w830:dbl)
                  n797 = global write "Global_count_var.vi" "Global count"(w830) -> ()
                }
              }
            }
            frame 3 {
              n798 = call "Forward.vi"("error in (no error)"=w834, "how close"=0.61) -> ("error out"=w835:errorcluster, "Done"=w836:bool)  [unwired: 8 in]
              n799 = case shown="True" w836 {
                frame False {
                }
                frame True {
                  n800 = global read "Stage_var.vi" "Stage"() -> (w842:u32)
                  n801 = global read "Global_count_var.vi" "Global count"() -> (w838:dbl)
                  n802 = call <vilib>:"High Resolution Relative Seconds.vi"() -> ("relative seconds"=w840:dbl)
                  n803 = Increment(x=w842) -> (x+1=w841:u32)
                  n804 = global write "Timer.vi" "Timer"(w840) -> ()
                  n805 = global write "Stage_var.vi" "Stage"(w841) -> ()
                  n806 = Increment(x=w838) -> (x+1=w839:dbl)
                  n807 = global write "Global_count_var.vi" "Global count"(w839) -> ()
                }
              }
            }
            frame 4 {
              n808 = call "Forward.vi"("error in (no error)"=w843, "how close"=0.8) -> ("error out"=w844:errorcluster, "Done"=w845:bool)  [unwired: 8 in]
              n809 = case shown="True" w845 {
                frame False {
                }
                frame True {
                  n810 = global read "Stage_var.vi" "Stage"() -> (w851:u32)
                  n811 = global read "Global_count_var.vi" "Global count"() -> (w847:dbl)
                  n812 = call <vilib>:"High Resolution Relative Seconds.vi"() -> ("relative seconds"=w849:dbl)
                  n813 = Increment(x=w851) -> (x+1=w850:u32)
                  n814 = global write "Timer.vi" "Timer"(w849) -> ()
                  n815 = global write "Stage_var.vi" "Stage"(w850) -> ()
                  n816 = Increment(x=w847) -> (x+1=w848:dbl)
                  n817 = global write "Global_count_var.vi" "Global count"(w848) -> ()
                }
              }
            }
            frame 5, Default {
              n818 = global write "Completed_var.vi" "Completed"(TRUE ("Completed")) -> ()
            }
            frame 1 {
              n819 = call "Forward.vi"("error in (no error)"=w857, "how close"=0.47) -> ("error out"=w856:errorcluster, "Done"=w854:bool)  [unwired: 8 in]
              n820 = case shown="True" w854 {
                frame False {
                }
                frame True {
                  n821 = global read "Stage_var.vi" "Stage"() -> (w862:u32)
                  n822 = call <vilib>:"High Resolution Relative Seconds.vi"() -> ("relative seconds"=w860:dbl)
                  n823 = global read "Global_count_var.vi" "Global count"() -> (w858:dbl)
                  n824 = Increment(x=w862) -> (x+1=w861:u32)
                  n825 = global write "Timer.vi" "Timer"(w860) -> ()
                  n826 = global write "Stage_var.vi" "Stage"(w861) -> ()
                  n827 = Increment(x=w858) -> (x+1=w859:dbl)
                  n828 = global write "Global_count_var.vi" "Global count"(w859) -> ()
                }
              }
            }
          }
        }
        frame 5 {
          n829 = global read "Ball_num_var.vi" "Ball num"() -> (w863:dbl)
          n830 = case shown="1" w863 {
            tunnel: w865 -> [w867 w880]
            tunnel: [w866 w879] -> w864
            frame Default {
              n831 = call "Rotation.vi"("error in (no error)"=w867, "Time"=2.8, "Direction"=90.0 ("how close")) -> ("error out"=w866:errorcluster, "Done"=w870:bool)  [unwired: 7 in]
              n832 = case shown="True" w870 {
                frame False {
                }
                frame True {
                  n833 = global read "Stage_var.vi" "Stage"() -> (w875:u32)
                  n834 = call <vilib>:"High Resolution Relative Seconds.vi"() -> ("relative seconds"=w873:dbl)
                  n835 = global read "Global_count_var.vi" "Global count"() -> (w871:dbl)
                  n836 = Increment(x=w875) -> (x+1=w874:u32)
                  n837 = global write "Timer.vi" "Timer"(w873) -> ()
                  n838 = global write "Stage_var.vi" "Stage"(w874) -> ()
                  n839 = Increment(x=w871) -> (x+1=w872:dbl)
                  n840 = global write "Global_count_var.vi" "Global count"(w872) -> ()
                }
              }
            }
            frame 1 {
              n841 = call "Rotation.vi"("error in (no error)"=w880, "Time"=2.8, "Direction"=-90.0 ("how close")) -> ("error out"=w879:errorcluster, "Done"=w878:bool)  [unwired: 7 in]
              n842 = case shown="True" w878 {
                frame False {
                }
                frame True {
                  n843 = global read "Global_count_var.vi" "Global count"() -> (w881:dbl)
                  n844 = global read "Stage_var.vi" "Stage"() -> (w885:u32)
                  n845 = call <vilib>:"High Resolution Relative Seconds.vi"() -> ("relative seconds"=w883:dbl)
                  n846 = Increment(x=w885) -> (x+1=w884:u32)
                  n847 = global write "Timer.vi" "Timer"(w883) -> ()
                  n848 = Increment(x=w881) -> (x+1=w882:dbl)
                  n849 = global write "Stage_var.vi" "Stage"(w884) -> ()
                  n850 = global write "Global_count_var.vi" "Global count"(w882) -> ()
                }
              }
            }
          }
        }
        frame 6 {
          n851 = global read "Sequence_var.vi" "Sequence"() -> (w907:dbl[])
          n852 = global read "Ball_num_var.vi" "Ball num"() -> (w891:dbl)
          n853 = Index Array(array=w907, index #1=0 ("index"), index #2=1 ("index"), index #3=2 ("index"), index #4=3 ("index")) -> (element #1=w902:dbl, element #2=w901:dbl, element #3=w900:dbl, element #4=w899:dbl)
          n854 = Equal?(x=w891, y=w902) -> (x = y?=w887:bool)
          n855 = Equal?(x=w891, y=w901) -> (x = y?=w888:bool)
          n856 = Equal?(x=w891, y=w900) -> (x = y?=w889:bool)
          n857 = Equal?(x=w891, y=w899) -> (x = y?=w890:bool)
          n858 = Build Array(w887, w888, w889, w890) -> (w886:bool[])
          n859 = Boolean Array To Number(Boolean array=w886) -> (number=w898:u32)
          n860 = call "Camera Motor Write.vi"("error in (no error)"=w896, "Camera Position (rad)"=-0.7) -> ("error out"=w894:errorcluster)  [unwired: 9 in]
          n861 = case shown="8" w898 {
            tunnel: ["Red" ("Combo Box") "Red" ("Combo Box") "Green" ("Combo Box") "Blue" ("Combo Box") "Yellow" ("Combo Box")] -> w897
            frame 0, Default {
            }
            frame 1 {
              n862 = global write "Color_num_var.vi" "Color now"(1.0 ("Color now")) -> ()
            }
            frame 2 {
              n863 = global write "Color_num_var.vi" "Color now"(2.0 ("Color now")) -> ()
            }
            frame 4 {
              n864 = global write "Color_num_var.vi" "Color now"(3.0 ("Color now")) -> ()
            }
            frame 8 {
              n865 = global write "Color_num_var.vi" "Color now"(4.0 ("Color now")) -> ()
            }
          }
          n866 = call "Take_it.vi"("error in (no error) 2"=w894, "Combo Box"=w897, "Camera Image"=w893) -> ("error out"=w908:errorcluster, "Done"=w892:bool)  [unwired: 7 in]
          n867 = case shown="True" w892 {
            frame False {
            }
            frame True {
              n868 = global read "Global_count_var.vi" "Global count"() -> (w909:dbl)
              n869 = global read "Stage_var.vi" "Stage"() -> (w913:u32)
              n870 = call <vilib>:"High Resolution Relative Seconds.vi"() -> ("relative seconds"=w911:dbl)
              n871 = Increment(x=w913) -> (x+1=w912:u32)
              n872 = Increment(x=w909) -> (x+1=w910:dbl)
              n873 = global write "Timer.vi" "Timer"(w911) -> ()
              n874 = global write "Stage_var.vi" "Stage"(w912) -> ()
              n875 = global write "Global_count_var.vi" "Global count"(w910) -> ()
            }
          }
        }
        frame 7 {
          n876 = global read "Ball_num_var.vi" "Ball num"() -> (w923:dbl)
          n877 = case shown="Default" w923 {
            tunnel: [w926 w937] -> w925
            tunnel: w924 -> [w927 w936]
            frame Default {
              n878 = call "Backward.vi"("error in (no error)"=w927, "how close"=0.47) -> ("error out"=w926:errorcluster, "Done"=w929:bool)  [unwired: 8 in]
              n879 = case shown="True" w929 {
                frame False {
                }
                frame True {
                  n880 = global read "Stage_var.vi" "Stage"() -> (w934:u32)
                  n881 = global read "Global_count_var.vi" "Global count"() -> (w930:dbl)
                  n882 = call <vilib>:"High Resolution Relative Seconds.vi"() -> ("relative seconds"=w932:dbl)
                  n883 = Increment(x=w934) -> (x+1=w933:u32)
                  n884 = global write "Timer.vi" "Timer"(w932) -> ()
                  n885 = global write "Stage_var.vi" "Stage"(w933) -> ()
                  n886 = Increment(x=w930) -> (x+1=w931:dbl)
                  n887 = global write "Global_count_var.vi" "Global count"(w931) -> ()
                }
              }
            }
            frame 1 {
              n888 = call "Backward.vi"("error in (no error)"=w936, "how close"=0.4) -> ("error out"=w937:errorcluster, "Done"=w938:bool)  [unwired: 8 in]
              n889 = case shown="True" w938 {
                frame False {
                }
                frame True {
                  n890 = global read "Global_count_var.vi" "Global count"() -> (w939:dbl)
                  n891 = global read "Stage_var.vi" "Stage"() -> (w943:u32)
                  n892 = call <vilib>:"High Resolution Relative Seconds.vi"() -> ("relative seconds"=w941:dbl)
                  n893 = Increment(x=w943) -> (x+1=w942:u32)
                  n894 = global write "Timer.vi" "Timer"(w941) -> ()
                  n895 = global write "Stage_var.vi" "Stage"(w942) -> ()
                  n896 = Increment(x=w939) -> (x+1=w940:dbl)
                  n897 = global write "Global_count_var.vi" "Global count"(w940) -> ()
                }
              }
            }
          }
        }
        frame 8 {
          n898 = global read "Ball_num_var.vi" "Ball num"() -> (w944:dbl)
          n899 = case shown="1" w944 {
            tunnel: w946 -> [w948 w958]
            tunnel: [w947 w957] -> w945
            frame Default {
              n900 = call "Rotation.vi"("error in (no error)"=w948, "Time"=3.0, "Direction"=90.0 ("how close")) -> ("error out"=w947:errorcluster, "Done"=w951:bool)  [unwired: 7 in]
              n901 = case shown="True" w951 {
                frame False {
                }
                frame True {
                  n902 = global read "Stage_var.vi" "Stage"() -> (w956:u32)
                  n903 = call <vilib>:"High Resolution Relative Seconds.vi"() -> ("relative seconds"=w954:dbl)
                  n904 = global read "Global_count_var.vi" "Global count"() -> (w952:dbl)
                  n905 = Increment(x=w956) -> (x+1=w955:u32)
                  n906 = global write "Timer.vi" "Timer"(w954) -> ()
                  n907 = global write "Stage_var.vi" "Stage"(w955) -> ()
                  n908 = Increment(x=w952) -> (x+1=w953:dbl)
                  n909 = global write "Global_count_var.vi" "Global count"(w953) -> ()
                }
              }
            }
            frame 1 {
              n910 = call "Rotation.vi"("error in (no error)"=w958, "Time"=4.9, "Direction"=-90.0 ("how close")) -> ("error out"=w957:errorcluster, "Done"=w961:bool)  [unwired: 7 in]
              n911 = case shown="True" w961 {
                frame False {
                }
                frame True {
                  n912 = global read "Global_count_var.vi" "Global count"() -> (w962:dbl)
                  n913 = global read "Stage_var.vi" "Stage"() -> (w966:u32)
                  n914 = call <vilib>:"High Resolution Relative Seconds.vi"() -> ("relative seconds"=w964:dbl)
                  n915 = Increment(x=w966) -> (x+1=w965:u32)
                  n916 = global write "Timer.vi" "Timer"(w964) -> ()
                  n917 = global write "Stage_var.vi" "Stage"(w965) -> ()
                  n918 = Increment(x=w962) -> (x+1=w963:dbl)
                  n919 = global write "Global_count_var.vi" "Global count"(w963) -> ()
                }
              }
            }
          }
        }
        frame 9 {
          # "Едем с первым шариком"
          n920 = call "Forward.vi"("error in (no error)"=w968, "how close"=0.18) -> ("error out"=w967:errorcluster, "Done"=w969:bool)  [unwired: 8 in]
          n921 = case shown="True" w969 {
            frame False {
            }
            frame True {
              n922 = global read "Stage_var.vi" "Stage"() -> (w975:u32)
              n923 = global read "Global_count_var.vi" "Global count"() -> (w971:dbl)
              n924 = call <vilib>:"High Resolution Relative Seconds.vi"() -> ("relative seconds"=w973:dbl)
              n925 = Increment(x=w975) -> (x+1=w974:u32)
              n926 = global write "Timer.vi" "Timer"(w973) -> ()
              n927 = global write "Stage_var.vi" "Stage"(w974) -> ()
              n928 = Increment(x=w971) -> (x+1=w972:dbl)
              n929 = global write "Global_count_var.vi" "Global count"(w972) -> ()
            }
          }
        }
        frame 10 {
          n930 = call "Rotation.vi"("error in (no error)"=w977, "Time"=3.2, "Direction"=90.0 ("how close")) -> ("error out"=w976:errorcluster, "Done"=w980:bool)  [unwired: 7 in]
          n931 = case shown="True" w980 {
            frame False {
            }
            frame True {
              n932 = global read "Stage_var.vi" "Stage"() -> (w985:u32)
              n933 = call <vilib>:"High Resolution Relative Seconds.vi"() -> ("relative seconds"=w983:dbl)
              n934 = global read "Global_count_var.vi" "Global count"() -> (w981:dbl)
              n935 = Increment(x=w985) -> (x+1=w984:u32)
              n936 = global write "Timer.vi" "Timer"(w983) -> ()
              n937 = global write "Stage_var.vi" "Stage"(w984) -> ()
              n938 = Increment(x=w981) -> (x+1=w982:dbl)
              n939 = global write "Global_count_var.vi" "Global count"(w982) -> ()
            }
          }
        }
        frame 11 {
          # "Едем до контрольной"
          n940 = call "Forward.vi"("error in (no error)"=w986, "how close"=0.45) -> ("error out"=w987:errorcluster, "Done"=w988:bool)  [unwired: 8 in]
          n941 = case shown="True" w988 {
            frame False {
            }
            frame True {
              n942 = global read "Global_count_var.vi" "Global count"() -> (w990:dbl)
              n943 = global read "Stage_var.vi" "Stage"() -> (w994:u32)
              n944 = call <vilib>:"High Resolution Relative Seconds.vi"() -> ("relative seconds"=w992:dbl)
              n945 = Increment(x=w994) -> (x+1=w993:u32)
              n946 = global write "Timer.vi" "Timer"(w992) -> ()
              n947 = Increment(x=w990) -> (x+1=w991:dbl)
              n948 = global write "Stage_var.vi" "Stage"(w993) -> ()
              n949 = global write "Global_count_var.vi" "Global count"(w991) -> ()
            }
          }
        }
        frame 12 {
          # "Поворот на контрольной"
          n950 = call "Rotation.vi"("error in (no error)"=w996, "Time"=3.0, "Direction"=90.0 ("how close")) -> ("error out"=w995:errorcluster, "Done"=w999:bool)  [unwired: 7 in]
          n951 = case shown="True" w999 {
            frame False {
            }
            frame True {
              n952 = global read "Stage_var.vi" "Stage"() -> (w1004:u32)
              n953 = global read "Global_count_var.vi" "Global count"() -> (w1000:dbl)
              n954 = call <vilib>:"High Resolution Relative Seconds.vi"() -> ("relative seconds"=w1002:dbl)
              n955 = Increment(x=w1004) -> (x+1=w1003:u32)
              n956 = global write "Timer.vi" "Timer"(w1002) -> ()
              n957 = global write "Stage_var.vi" "Stage"(w1003) -> ()
              n958 = Increment(x=w1000) -> (x+1=w1001:dbl)
              n959 = global write "Global_count_var.vi" "Global count"(w1001) -> ()
            }
          }
        }
        frame Default {
        }
      }
      n960 = case shown="3" w90 {
        tunnel: w93 -> [w1036 w1106 w1171 w1246 w1318]
        tunnel: [w1046 w1105 w1169 w1244 w1319] -> w97
        tunnel: w94 -> [w1018 w1092 w1167 w1242 w1319]
        tunnel: [w1035 w1104 w1170 w1245 w1318] -> _
        tunnel: w91 -> [w1017 w1093 w1168 w1243 _]
        frame 0 {
          w1048 = u16 2 items=["RGB", "HSL", "HSV", "HSI"] ("Color Mode")
          n961 = call "IMAQ ColorThreshold"("Blue or Luma or Val or Inten Range"=cluster{"Lower value":i32, "Upper value":i32} {"Lower value"=0, "Upper value"=255} ("Red or Hue Range"), "Replace Value"=255, "Green or Sat Range"=cluster{"Lower value":i32, "Upper value":i32} {"Lower value"=80, "Upper value"=255} ("Red or Hue Range"), "Color Mode"=w1048, "error in (no error)"=w1018, "Red or Hue Range"=cluster{"Lower value":i32, "Upper value":i32} {"Lower value"=0, "Upper value"=30}, "Image Dst"=w1036, "Image Src"=w1017) -> ("error out"=w1053:errorcluster, "Image Dst Out"=w1035:T1)  [unwired: 2 in]
          n962 = call "IMAQ Centroid"("error in (no error)"=w1053, "Image Mask"=w1035, "Image"=w1036) -> ("error out"=w1052:errorcluster, "Centroid"=w1026:cluster{"X Centroid":sgl, "Y Centroid":sgl})  [unwired: 1 in]
          n963 = global read "Sequence_var.vi" "Sequence"() -> (w1021:dbl[])
          n964 = Unbundle By Name(w1026) -> ("X Centroid"=w1045:sgl)
          n965 = Unbundle By Name(w1026) -> ("X Centroid"=w1029:sgl)
          n966 = Unbundle By Name(w1026) -> ("X Centroid"=w1033:sgl)
          n967 = Unbundle By Name(w1026) -> ("X Centroid"=w1041:sgl)
          n968 = Unbundle By Name(w1026) -> ("X Centroid"=w1039:sgl)
          n969 = Merge Errors(w1052, w1053) -> (w1046:errorcluster)
          n970 = Index Array(array=w1021, index=0) -> (element=w1020:dbl)
          n971 = Less?(x=w1045, y=sgl 110.0) -> (x < y?=w1043:bool)
          n972 = Greater Or Equal?(x=w1029, y=sgl 110.0) -> (x >= y?=w1030:bool)
          n973 = Less?(x=w1033, y=sgl 255.0) -> (x < y?=w1032:bool)
          n974 = Greater Or Equal?(x=w1041, y=sgl 255.0) -> (x >= y?=w1040:bool)
          n975 = Equal?(x=w1039, y=sgl 160.0) -> (x = y?=w1037:bool)
          n976 = Not Equal?(x=sgl 160.0 ("y"), y=w1029) -> (x != y?=w1027:bool)
          n977 = And(x=w1030, y=w1032) -> (x .and. y?=w1024:bool)
          n978 = And(x=w1027, y=w1024) -> (x .and. y?=w1025:bool)
          n979 = Not Equal?(x=w1020, y=0.0) -> (x != y?=w1023:bool)
          n980 = case shown="True" w1037 {
            frame False {
            }
            frame True {
              n981 = global read "Sequence_var.vi" "Sequence"() -> (w1064:dbl[])
              n982 = Index Array(array=w1064, index #1=1 ("index"), index #2=2 ("index"), index #3=3 ("index")) -> (element #1=w1058:dbl, element #2=w1059:dbl, element #3=w1060:dbl)
              n983 = Build Array(1.0 ("element"), w1058, w1059, w1060) -> (w1056:dbl[])
              n984 = global write "Sequence_var.vi" "Sequence"(w1056) -> ()
            }
          }
          n985 = case shown="True" w1025 {
            frame False {
            }
            frame True {
              n986 = global read "Sequence_var.vi" "Sequence"() -> (w1073:dbl[])
              n987 = Index Array(array=w1073, index #1=1 ("index"), index #2=2 ("index"), index #3=3 ("index")) -> (element #1=w1067:dbl, element #2=w1068:dbl, element #3=w1069:dbl)
              n988 = Build Array(3.0 ("element"), w1067, w1068, w1069) -> (w1065:dbl[])
              n989 = global write "Sequence_var.vi" "Sequence"(w1065) -> ()
            }
          }
          n990 = case shown="True" w1040 {
            frame False {
            }
            frame True {
              n991 = global read "Sequence_var.vi" "Sequence"() -> (w1082:dbl[])
              n992 = Index Array(array=w1082, index #1=1 ("index"), index #2=2 ("index"), index #3=3 ("index")) -> (element #1=w1076:dbl, element #2=w1077:dbl, element #3=w1078:dbl)
              n993 = Build Array(4.0 ("element"), w1076, w1077, w1078) -> (w1074:dbl[])
              n994 = global write "Sequence_var.vi" "Sequence"(w1074) -> ()
            }
          }
          n995 = case shown="True" w1043 {
            frame False {
            }
            frame True {
              n996 = global read "Sequence_var.vi" "Sequence"() -> (w1091:dbl[])
              n997 = Index Array(array=w1091, index #1=1 ("index"), index #2=2 ("index"), index #3=3 ("index")) -> (element #1=w1085:dbl, element #2=w1086:dbl, element #3=w1087:dbl)
              n998 = Build Array(2.0 ("element"), w1085, w1086, w1087) -> (w1083:dbl[])
              n999 = global write "Sequence_var.vi" "Sequence"(w1083) -> ()
            }
          }
          n1000 = case shown="True" w1023 {
            frame False {
            }
            frame True {
              n1001 = global read "Stage_var.vi" "Stage"() -> (w1055:u32)
              n1002 = Increment(x=w1055) -> (x+1=w1054:u32)
              n1003 = global write "Stage_var.vi" "Stage"(w1054) -> ()
            }
          }
        }
        frame 1 {
          w1123 = u16 2 items=["RGB", "HSL", "HSV", "HSI"] ("Color Mode")
          n1004 = call "IMAQ ColorThreshold"("Blue or Luma or Val or Inten Range"=cluster{"Lower value":i32, "Upper value":i32} {"Lower value"=0, "Upper value"=255} ("Red or Hue Range"), "Replace Value"=255, "Green or Sat Range"=cluster{"Lower value":i32, "Upper value":i32} {"Lower value"=0, "Upper value"=255} ("Red or Hue Range"), "Color Mode"=w1123, "error in (no error)"=w1092, "Red or Hue Range"=cluster{"Lower value":i32, "Upper value":i32} {"Lower value"=55, "Upper value"=100}, "Image Dst"=w1106, "Image Src"=w1093) -> ("error out"=w1128:errorcluster, "Image Dst Out"=w1104:T1)  [unwired: 2 in]
          n1005 = call "IMAQ Centroid"("error in (no error)"=w1128, "Image Mask"=w1104, "Image"=w1106) -> ("error out"=w1127:errorcluster, "Centroid"=w1110:cluster{"X Centroid":sgl, "Y Centroid":sgl})  [unwired: 1 in]
          n1006 = global read "Sequence_var.vi" "Sequence"() -> (w1096:dbl[])
          n1007 = Unbundle By Name(w1110) -> ("X Centroid"=w1121:sgl)
          n1008 = Unbundle By Name(w1110) -> ("X Centroid"=w1117:sgl)
          n1009 = Unbundle By Name(w1110) -> ("X Centroid"=w1103:sgl)
          n1010 = Unbundle By Name(w1110) -> ("X Centroid"=w1114:sgl)
          n1011 = Unbundle By Name(w1110) -> ("X Centroid"=w1109:sgl)
          n1012 = Merge Errors(w1127, w1128) -> (w1105:errorcluster)
          n1013 = Index Array(array=w1096, index=1) -> (element=w1095:dbl)
          n1014 = Less?(x=w1121, y=sgl 110.0) -> (x < y?=w1119:bool)
          n1015 = Greater Or Equal?(x=w1117, y=sgl 250.0) -> (x >= y?=w1116:bool)
          n1016 = Greater Or Equal?(x=w1103, y=sgl 110.0) -> (x >= y?=w1111:bool)
          n1017 = Less?(x=w1114, y=sgl 250.0) -> (x < y?=w1113:bool)
          n1018 = Equal?(x=w1109, y=sgl 160.0) -> (x = y?=w1107:bool)
          n1019 = Not Equal?(x=sgl 160.0 ("y"), y=w1103) -> (x != y?=w1100:bool)
          n1020 = Not Equal?(x=w1095, y=0.0) -> (x != y?=w1098:bool)
          n1021 = And(x=w1111, y=w1113) -> (x .and. y?=w1099:bool)
          n1022 = And(x=w1100, y=w1099) -> (x .and. y?=w1101:bool)
          n1023 = case shown="True" w1107 {
            frame False {
            }
            frame True {
              n1024 = global read "Sequence_var.vi" "Sequence"() -> (w1139:dbl[])
              n1025 = Index Array(array=w1139, index #1=0 ("index"), index #2=2 ("index"), index #3=3 ("index")) -> (element #1=w1132:dbl, element #2=w1134:dbl, element #3=w1135:dbl)
              n1026 = Build Array(w1132, 1.0 ("element"), w1134, w1135) -> (w1133:dbl[])
              n1027 = global write "Sequence_var.vi" "Sequence"(w1133) -> ()
            }
          }
          n1028 = case shown="True" w1101 {
            frame False {
            }
            frame True {
              n1029 = global read "Sequence_var.vi" "Sequence"() -> (w1148:dbl[])
              n1030 = Index Array(array=w1148, index #1=0 ("index"), index #2=2 ("index"), index #3=3 ("index")) -> (element #1=w1141:dbl, element #2=w1143:dbl, element #3=w1144:dbl)
              n1031 = Build Array(w1141, 3.0 ("element"), w1143, w1144) -> (w1142:dbl[])
              n1032 = global write "Sequence_var.vi" "Sequence"(w1142) -> ()
            }
          }
          n1033 = case shown="True" w1116 {
            frame False {
            }
            frame True {
              n1034 = global read "Sequence_var.vi" "Sequence"() -> (w1157:dbl[])
              n1035 = Index Array(array=w1157, index #1=0 ("index"), index #2=2 ("index"), index #3=3 ("index")) -> (element #1=w1149:dbl, element #2=w1152:dbl, element #3=w1153:dbl)
              n1036 = Build Array(w1149, 4.0 ("element"), w1152, w1153) -> (w1151:dbl[])
              n1037 = global write "Sequence_var.vi" "Sequence"(w1151) -> ()
            }
          }
          n1038 = case shown="True" w1119 {
            frame False {
            }
            frame True {
              n1039 = global read "Sequence_var.vi" "Sequence"() -> (w1166:dbl[])
              n1040 = Index Array(array=w1166, index #1=0 ("index"), index #2=2 ("index"), index #3=3 ("index")) -> (element #1=w1158:dbl, element #2=w1161:dbl, element #3=w1162:dbl)
              n1041 = Build Array(w1158, 2.0 ("element"), w1161, w1162) -> (w1160:dbl[])
              n1042 = global write "Sequence_var.vi" "Sequence"(w1160) -> ()
            }
          }
          n1043 = case shown="True" w1098 {
            frame False {
            }
            frame True {
              n1044 = global read "Stage_var.vi" "Stage"() -> (w1130:u32)
              n1045 = Increment(x=w1130) -> (x+1=w1129:u32)
              n1046 = global write "Stage_var.vi" "Stage"(w1129) -> ()
            }
          }
        }
        frame 2 {
          w1198 = u16 2 items=["RGB", "HSL", "HSV", "HSI"] ("Color Mode")
          n1047 = call "IMAQ ColorThreshold"("Blue or Luma or Val or Inten Range"=cluster{"Lower value":i32, "Upper value":i32} {"Lower value"=0, "Upper value"=255} ("Red or Hue Range"), "Replace Value"=255, "Green or Sat Range"=cluster{"Lower value":i32, "Upper value":i32} {"Lower value"=0, "Upper value"=255} ("Red or Hue Range"), "Color Mode"=w1198, "error in (no error)"=w1167, "Red or Hue Range"=cluster{"Lower value":i32, "Upper value":i32} {"Lower value"=130, "Upper value"=220}, "Image Dst"=w1171, "Image Src"=w1168) -> ("error out"=w1203:errorcluster, "Image Dst Out"=w1170:T1)  [unwired: 2 in]
          n1048 = call "IMAQ Centroid"("error in (no error)"=w1203, "Image Mask"=w1170, "Image"=w1171) -> ("error out"=w1202:errorcluster, "Centroid"=w1185:cluster{"X Centroid":sgl, "Y Centroid":sgl})  [unwired: 1 in]
          n1049 = global read "Sequence_var.vi" "Sequence"() -> (w1174:dbl[])
          n1050 = Unbundle By Name(w1185) -> ("X Centroid"=w1196:sgl)
          n1051 = Unbundle By Name(w1185) -> ("X Centroid"=w1192:sgl)
          n1052 = Unbundle By Name(w1185) -> ("X Centroid"=w1181:sgl)
          n1053 = Unbundle By Name(w1185) -> ("X Centroid"=w1189:sgl)
          n1054 = Unbundle By Name(w1185) -> ("X Centroid"=w1184:sgl)
          n1055 = Merge Errors(w1202, w1203) -> (w1169:errorcluster)
          n1056 = Index Array(array=w1174, index=2) -> (element=w1173:dbl)
          n1057 = Less?(x=w1196, y=sgl 110.0) -> (x < y?=w1194:bool)
          n1058 = Greater Or Equal?(x=w1192, y=sgl 250.0) -> (x >= y?=w1191:bool)
          n1059 = Greater Or Equal?(x=w1181, y=sgl 110.0) -> (x >= y?=w1186:bool)
          n1060 = Less?(x=w1189, y=sgl 250.0) -> (x < y?=w1188:bool)
          n1061 = Equal?(x=w1184, y=sgl 160.0) -> (x = y?=w1182:bool)
          n1062 = Not Equal?(x=sgl 160.0 ("y"), y=w1181) -> (x != y?=w1178:bool)
          n1063 = Not Equal?(x=w1173, y=0.0) -> (x != y?=w1176:bool)
          n1064 = And(x=w1186, y=w1188) -> (x .and. y?=w1177:bool)
          n1065 = And(x=w1178, y=w1177) -> (x .and. y?=w1179:bool)
          n1066 = case shown="True" w1182 {
            frame False {
            }
            frame True {
              n1067 = global read "Sequence_var.vi" "Sequence"() -> (w1214:dbl[])
              n1068 = Index Array(array=w1214, index #1=0 ("index"), index #2=1 ("index"), index #3=3 ("index")) -> (element #1=w1206:dbl, element #2=w1207:dbl, element #3=w1210:dbl)
              n1069 = Build Array(w1206, w1207, 1.0 ("element"), w1210) -> (w1209:dbl[])
              n1070 = global write "Sequence_var.vi" "Sequence"(w1209) -> ()
            }
          }
          n1071 = case shown="True" w1179 {
            frame False {
            }
            frame True {
              n1072 = global read "Sequence_var.vi" "Sequence"() -> (w1223:dbl[])
              n1073 = Index Array(array=w1223, index #1=0 ("index"), index #2=1 ("index"), index #3=3 ("index")) -> (element #1=w1215:dbl, element #2=w1216:dbl, element #3=w1219:dbl)
              n1074 = Build Array(w1215, w1216, 3.0 ("element"), w1219) -> (w1218:dbl[])
              n1075 = global write "Sequence_var.vi" "Sequence"(w1218) -> ()
            }
          }
          n1076 = case shown="True" w1191 {
            frame False {
            }
            frame True {
              n1077 = global read "Sequence_var.vi" "Sequence"() -> (w1232:dbl[])
              n1078 = Index Array(array=w1232, index #1=0 ("index"), index #2=1 ("index"), index #3=3 ("index")) -> (element #1=w1224:dbl, element #2=w1225:dbl, element #3=w1228:dbl)
              n1079 = Build Array(w1224, w1225, 4.0 ("element"), w1228) -> (w1227:dbl[])
              n1080 = global write "Sequence_var.vi" "Sequence"(w1227) -> ()
            }
          }
          n1081 = case shown="True" w1194 {
            frame False {
            }
            frame True {
              n1082 = global read "Sequence_var.vi" "Sequence"() -> (w1241:dbl[])
              n1083 = Index Array(array=w1241, index #1=0 ("index"), index #2=1 ("index"), index #3=3 ("index")) -> (element #1=w1233:dbl, element #2=w1234:dbl, element #3=w1237:dbl)
              n1084 = Build Array(w1233, w1234, 2.0 ("element"), w1237) -> (w1236:dbl[])
              n1085 = global write "Sequence_var.vi" "Sequence"(w1236) -> ()
            }
          }
          n1086 = case shown="True" w1176 {
            frame False {
            }
            frame True {
              n1087 = global read "Stage_var.vi" "Stage"() -> (w1205:u32)
              n1088 = Increment(x=w1205) -> (x+1=w1204:u32)
              n1089 = global write "Stage_var.vi" "Stage"(w1204) -> ()
            }
          }
        }
        frame 3 {
          w1273 = u16 2 items=["RGB", "HSL", "HSV", "HSI"] ("Color Mode")
          n1090 = call "IMAQ ColorThreshold"("Blue or Luma or Val or Inten Range"=cluster{"Lower value":i32, "Upper value":i32} {"Lower value"=0, "Upper value"=255} ("Red or Hue Range"), "Replace Value"=255, "Green or Sat Range"=cluster{"Lower value":i32, "Upper value":i32} {"Lower value"=0, "Upper value"=255} ("Red or Hue Range"), "Color Mode"=w1273, "error in (no error)"=w1242, "Red or Hue Range"=cluster{"Lower value":i32, "Upper value":i32} {"Lower value"=25, "Upper value"=50}, "Image Dst"=w1246, "Image Src"=w1243) -> ("error out"=w1278:errorcluster, "Image Dst Out"=w1245:T1)  [unwired: 2 in]
          n1091 = call "IMAQ Centroid"("error in (no error)"=w1278, "Image Mask"=w1245, "Image"=w1246) -> ("error out"=w1277:errorcluster, "Centroid"=w1260:cluster{"X Centroid":sgl, "Y Centroid":sgl})  [unwired: 1 in]
          n1092 = global read "Sequence_var.vi" "Sequence"() -> (w1249:dbl[])
          n1093 = Unbundle By Name(w1260) -> ("X Centroid"=w1271:sgl)
          n1094 = Unbundle By Name(w1260) -> ("X Centroid"=w1267:sgl)
          n1095 = Unbundle By Name(w1260) -> ("X Centroid"=w1256:sgl)
          n1096 = Unbundle By Name(w1260) -> ("X Centroid"=w1264:sgl)
          n1097 = Unbundle By Name(w1260) -> ("X Centroid"=w1259:sgl)
          n1098 = Merge Errors(w1277, w1278) -> (w1244:errorcluster)
          n1099 = Index Array(array=w1249, index=3) -> (element=w1248:dbl)
          n1100 = Less?(x=w1271, y=sgl 110.0) -> (x < y?=w1269:bool)
          n1101 = Greater Or Equal?(x=w1267, y=sgl 250.0) -> (x >= y?=w1266:bool)
          n1102 = Greater Or Equal?(x=w1256, y=sgl 110.0) -> (x >= y?=w1261:bool)
          n1103 = Less?(x=w1264, y=sgl 250.0) -> (x < y?=w1263:bool)
          n1104 = Equal?(x=w1259, y=sgl 160.0) -> (x = y?=w1257:bool)
          n1105 = Not Equal?(x=sgl 160.0 ("y"), y=w1256) -> (x != y?=w1253:bool)
          n1106 = Not Equal?(x=w1248, y=0.0) -> (x != y?=w1251:bool)
          n1107 = And(x=w1261, y=w1263) -> (x .and. y?=w1252:bool)
          n1108 = And(x=w1253, y=w1252) -> (x .and. y?=w1254:bool)
          n1109 = case shown="True" w1257 {
            frame False {
            }
            frame True {
              n1110 = global read "Sequence_var.vi" "Sequence"() -> (w1290:dbl[])
              n1111 = Index Array(array=w1290, index #1=0 ("index"), index #2=1 ("index"), index #3=2 ("index")) -> (element #1=w1282:dbl, element #2=w1283:dbl, element #3=w1284:dbl)
              n1112 = Build Array(w1282, w1283, w1284, 1.0 ("element")) -> (w1286:dbl[])
              n1113 = global write "Sequence_var.vi" "Sequence"(w1286) -> ()
            }
          }
          n1114 = case shown="True" w1254 {
            frame False {
            }
            frame True {
              n1115 = global read "Sequence_var.vi" "Sequence"() -> (w1299:dbl[])
              n1116 = Index Array(array=w1299, index #1=0 ("index"), index #2=1 ("index"), index #3=2 ("index")) -> (element #1=w1294:dbl, element #2=w1293:dbl, element #3=w1292:dbl)
              n1117 = Build Array(w1294, w1293, w1292, 3.0 ("element")) -> (w1295:dbl[])
              n1118 = global write "Sequence_var.vi" "Sequence"(w1295) -> ()
            }
          }
          n1119 = case shown="True" w1266 {
            frame False {
            }
            frame True {
              n1120 = global read "Sequence_var.vi" "Sequence"() -> (w1308:dbl[])
              n1121 = Index Array(array=w1308, index #1=0 ("index"), index #2=1 ("index"), index #3=2 ("index")) -> (element #1=w1302:dbl, element #2=w1301:dbl, element #3=w1300:dbl)
              n1122 = Build Array(w1302, w1301, w1300, 4.0 ("element")) -> (w1304:dbl[])
              n1123 = global write "Sequence_var.vi" "Sequence"(w1304) -> ()
            }
          }
          n1124 = case shown="True" w1269 {
            frame False {
            }
            frame True {
              n1125 = global read "Sequence_var.vi" "Sequence"() -> (w1317:dbl[])
              n1126 = Index Array(array=w1317, index #1=0 ("index"), index #2=1 ("index"), index #3=2 ("index")) -> (element #1=w1312:dbl, element #2=w1311:dbl, element #3=w1310:dbl)
              n1127 = Build Array(w1312, w1311, w1310, 2.0 ("element")) -> (w1313:dbl[])
              n1128 = global write "Sequence_var.vi" "Sequence"(w1313) -> ()
            }
          }
          n1129 = case shown="True" w1251 {
            frame False {
            }
            frame True {
              n1130 = global read "Stage_var.vi" "Stage"() -> (w1281:u32)
              n1131 = global write "Scanned.vi" "Scanned"(TRUE ("Scanned")) -> ()
              n1132 = Increment(x=w1281) -> (x+1=w1280:u32)
              n1133 = global write "Stage_var.vi" "Stage"(w1280) -> ()
            }
          }
        }
        frame Default {
        }
      }
      n1134 = Merge Errors(w97, w96, w89) -> (w95:errorcluster)
    }
  }
  "error out" <- w75
  n1135 = global read "Scanned.vi" "Scanned"() -> (w35:bool)
  "Scanned" <- w35
  n1136 = Boolean To (0,1)(Boolean=w35) -> (0, 1=w34:i16)
  n1137 = global read "Arm_stage_var.vi" "Arm stage"() -> (→"Arm stage":dbl)
  n1138 = global read "Completed_var.vi" "Completed"() -> (→"Completed":bool)
  n1139 = Number To Decimal String(number=w34) -> (decimal integer string=w33:string)  [unwired: 1 in]
  n1140 = Concatenate Strings(w10, "/" ("string"), w33) -> (w25:string)
  n1141 = global read "Sequence_var.vi" "Sequence"() -> (w32:dbl[])
  "Sequence" <- w32
  n1142 = Index Array(array=w32, index #1=0 ("index"), index #2=1 ("index"), index #3=2 ("index"), index #4=3 ("index")) -> (element #1=w23:dbl, element #2=w19:dbl, element #3=w15:dbl, element #4=w11:dbl)
  n1143 = Number To Decimal String(number=w23) -> (decimal integer string=w24:string)  [unwired: 1 in]
  n1144 = Concatenate Strings(w25, "/" ("string"), w24) -> (w20:string)
  n1145 = global read "Global_count_var.vi" "Global count"() -> (w6:dbl)
  "Performing..." <- w6
  "Stage" <- w6
  n1146 = Number To Decimal String(number=w19) -> (decimal integer string=w22:string)  [unwired: 1 in]
  n1147 = Concatenate Strings(w20, "/" ("string"), w22) -> (w16:string)
  n1148 = Number To Decimal String(number=w15) -> (decimal integer string=w17:string)  [unwired: 1 in]
  n1149 = Concatenate Strings(w16, "/" ("string"), w17) -> (w12:string)
  n1150 = Number To Decimal String(number=w11) -> (decimal integer string=w14:string)  [unwired: 1 in]
  n1151 = Concatenate Strings(w12, "/" ("string"), w14) -> (w7:string)
  n1152 = Number To Decimal String(number=w6) -> (decimal integer string=w8:string)  [unwired: 1 in]
  n1153 = Concatenate Strings(w7, "/" ("string"), w8) -> (w3:string)
  n1154 = global read "Ball_num_var.vi" "Ball num"() -> (w2:dbl)
  "Ball num" <- w2
  n1155 = Number To Decimal String(number=w2) -> (decimal integer string=w5:string)  [unwired: 1 in]
  n1156 = Concatenate Strings(w3, "/" ("string"), w5) -> (→"data out":string)
